vi "Ballistics_PBBA_beta.vi"() -> ()   [LabVIEW 2012]
doc: "This program is currently beta software. It is designed to address the data requirements defined primarily by the DHB Ballistic Test Report.\n\nThe general operation of this program is based on the Ballistics Version 2005 application developed internally by DuPont as a research tool for the Spruance Plant Ballistics Lab in Richmond, VA.\n\nPlease note that the original trigger control logic was modified and no longer depends on a safety interlock system to enable operation of a ballistic test.\n\nDuPont makes no warranties and assumes no liabilities in connection with any use of this program."
uses:
  <vilib>/Utility/NIReport.llb/NI_report.lvclass
  <vilib>/addons/database/NI_Database_API.lvlib
  <vilib>/addons/database/Connection.llb/Conn Execute.vi
  <vilib>/addons/database/Recordset.llb/Rec Destroy - Connection.vi
  <vilib>/Utility/config.llb/NI_LVConfig.lvlib
  <vilib>/Utility/config.llb/Write Key (I32).vi
  <vilib>/Analysis/NI_AALBase.lvlib
  Instance           1 28Saved   Ballistics_PBBA_beta .vi
  Shot Record.ctl
  <vilib>/addons/database/Connection.llb/DB Tools Open Connec (String).vi
  <vilib>/Utility/NIReport.llb/Append Text Table to Report (wrap).vi
  <vilib>/Utility/NIReport.llb/Append Report Text (str wrap).vi
panel:
  in  "RESET All":bool
  in  "EXIT":bool
  in  "Stop Program":bool
  in  "mainTabCntrl":enum32{"SETUP", "MEASURE", "HISTORY", "ABOUT"}(tab)
  in  "setupTabCntrl":T1(tab)
  in  "Model":u16(ring) caption="Model #" items=["n/a", "undefined", "other"]
  in  "clayCalArray":i16[](array[numeric])=[0, 0, 0, 0, 0] caption="Calibration" min=0 max=99 format="%02.0f"
  in  "Panel Dimensions":u16(ring)=6 caption="Panel Size" items=["7.5x7.5", "8.5x11", "12X12", "12x15", "13X13", "15X16", "15x15", "15x18", "16X16", "18X18", "20X16", "24x24", "101/4x113/4", "26X26", "CHEST PLATE", "HELMET", "VEST PANEL", "n/a"]
  out "threatDetails":T2
  in  "projectileWt":u16(ring) caption="Weight (gr)" items=["Select . . .", "2", "4", "16", "17", "44", "45", "55", "62", "64", "85", "110", "115", "123", "124", "127", "148", "158", "166", "180", "207", "240"]
  out "clayAverage":sgl caption="Clay Average" format="%#.1f"
  in  "clayTemp":i16 caption="Clay Temperature"
  in  "RoomT":i32 caption="Room Temperature"
  in  "RoomHum":i32 caption="Room Humidity"
  in  "Sample #":string
  in  "Comments":string caption="Remark"
  in  "recorder":u16(ring) caption="Recorder" items=["Mike Slate", "Dan Kraus", "Pat Fitzgerald", "Other"]
  in  "shooter":u16(ring) caption="Shooter" items=["Mike Slate", "Pat Fitzgerald", "Other"]
  in  "rangeNum":u16(ring) caption="Range #" items=["1", "2", "Other"]
  in  "projectileType":u16(ring) caption="Projectile Type"
  in  "weapon":u16(ring) caption="Weapon" items=["Universal Receiver", "Other"]
  in  "minV50":i32=1500 caption="Min. V50"
  in  "covering":u16(ring) caption="Ballistic Cover" items=["Other", "RipStop"]
  out "totalBAW":sgl caption="Total BAW" format="%.2f"
  in  "totalSampleWt":sgl caption="Total Weight" format="%.2f"
  in  "serialNum":string caption="Serial #"
  in  "workType":u16(ring) caption="Type of Work" items=["R&D", "QC", "Other"]
  in  "projNum":string caption="Project #"
  in  "projName":string caption="Project Name"
  in  "standard":u16(ring)=1 caption="Standard" items=["NIJ 0101.04", "MIL-STD-662F", "Other"]
  in  "Powder Type":u16(ring) items=["ACCURATE, NO. 2", "ACCURATE, NO. 9", "Alliant Herc. Bullseye", "Alliant 2400", "Hercules", "Hi-Skor 700x", "Hi-Skor 800x", "IMR-4198", "IMR-4756", "IMR-4895", "International Clay's", "Power Pistol", "Winchester Ball", "WINCHESTER-231", "WINCHESTER-296", "WINCHESTER-296"]
  in  "Method":u16(ring) items=["V50", "N.I.J.", "Quasi N.I.J.", "CUSUM", "V(0)", "V(0) @ 1450", "V(0) @ 1500", "V(0) @ 1550"]
  in  "Layer_1":T3={"plyNum"=0, "LotNum"="n/a", "RollNum"="n/a", "Fabric.stitch"=1} caption="Fabric #1" {"Fabric.stitch" items=["Corners", "Other", "n/a"]; "plyNum" min=0 max=99 step=5}
  in  "Layer_2":T3={"plyNum"=0, "LotNum"="n/a", "RollNum"="n/a", "Fabric.stitch"=1} caption="Fabric #2" {"Fabric.stitch" items=["Corners", "Other", "n/a"]; "plyNum" min=0 max=99 step=5}
  in  "Layer_3":T3={"plyNum"=0, "LotNum"="n/a", "RollNum"="n/a", "Fabric.stitch"=1} caption="Fabric #3" {"Fabric.stitch" items=["Corners", "Other", "n/a"]; "plyNum" min=0 max=99 step=5}
  in  "Layer_4":T3={"plyNum"=0, "LotNum"="n/a", "RollNum"="n/a", "Fabric.stitch"=1} caption="Fabric #4" {"Fabric.stitch" items=["Corners", "Other", "n/a"]; "plyNum" min=0 max=99 step=5}
  in  "Layer_5":T3={"plyNum"=0, "LotNum"="n/a", "RollNum"="n/a", "Fabric.stitch"=1} caption="Fabric #5" {"Fabric.stitch" items=["Corners", "Other", "n/a"]; "plyNum" min=0 max=99 step=5}
  in  "Layer_6":T3={"plyNum"=0, "LotNum"="n/a", "RollNum"="n/a", "Fabric.stitch"=1} caption="Fabric #6" {"Fabric.stitch" items=["Corners", "Other", "n/a"]; "plyNum" min=0 max=99 step=5}
  out "fabAttribs_1":T4 caption="fabricAttribs_1"
  out "fabAttribs_2":T4 caption="fabricAttribs_2"
  out "fabAttribs_3":T4 caption="fabricAttribs_3"
  out "fabAttribs_4":T4 caption="fabricAttribs_4"
  out "fabAttribs_5":T4 caption="fabricAttribs_5"
  out "fabAttribs_6":T4 caption="fabricAttribs_6"
  in  "fabStyle_1":u16(ring)
  in  "fabStyle_2":u16(ring)
  in  "fabStyle_3":u16(ring)
  in  "fabStyle_4":u16(ring)
  in  "fabStyle_5":u16(ring)
  in  "fabStyle_6":u16(ring)
  in  "fabVendor_1":u16(ring) caption="vendor" items=[" Select Vendor . . .", "Barrday", "Cushman", "DSM", "FMS", "Hexcell", "Honeywell", "Lincoln", "Pro Systems", "TEIJIN", "TexTech"]
  in  "fabVendor_2":u16(ring) caption="vendor" items=[" Select Vendor . . .", "Barrday", "Cushman", "DSM", "FMS", "Hexcell", "Honeywell", "Lincoln", "Pro Systems", "TEIJIN", "TexTech"]
  in  "fabVendor_3":u16(ring) caption="vendor" items=[" Select Vendor . . .", "Barrday", "Cushman", "DSM", "FMS", "Hexcell", "Honeywell", "Lincoln", "Pro Systems", "TEIJIN", "TexTech"]
  in  "fabVendor_4":u16(ring) caption="vendor" items=[" Select Vendor . . .", "Barrday", "Cushman", "DSM", "FMS", "Hexcell", "Honeywell", "Lincoln", "Pro Systems", "TEIJIN", "TexTech"]
  in  "fabVendor_5":u16(ring) caption="vendor" items=[" Select Vendor . . .", "Barrday", "Cushman", "DSM", "FMS", "Hexcell", "Honeywell", "Lincoln", "Pro Systems", "TEIJIN", "TexTech"]
  in  "fabVendor_6":u16(ring) caption="vendor" items=[" Select Vendor . . .", "Barrday", "Cushman", "DSM", "FMS", "Hexcell", "Honeywell", "Lincoln", "Pro Systems", "TEIJIN", "TexTech"]
  out "fab6_totalWt":sgl caption="Fab6 Wt" min=0 max=99 step=5 format="%.2f"
  out "fab5_totalWt":sgl caption="Fab5 Wt" min=0 max=99 step=5 format="%.2f"
  out "fab4_totalWt":sgl caption="Fab4 Wt" min=0 max=99 step=5 format="%.2f"
  out "fab3_totalWt":sgl caption="Fab3 Wt" min=0 max=99 step=5 format="%.2f"
  out "fab2_totalWt":sgl caption="Fab2 Wt" min=0 max=99 step=5 format="%.2f"
  out "fab1_totalWt":sgl caption="Fab1 Wt" min=0 max=99 step=5 format="%.2f"
  out "totalNumPlies":i32 caption="Total # of Plies" min=0 max=100 step=5
  in  "Next Shot":bool
  in  "Delete Button":bool
  in  "SHOTS":T5[](array[typedef]) {"UncorrectedAvgVel_PB" format="%.1f"; "strikeVel_PB" format="%.1f"; "velLoss_PB" format="%.1f"; "avgVel_PB" format="%.1f"; "Redundant_Velocity" format="%.1f"; "Energy Loss (J)" format="%.3e"; "Projectile Mass" min=0 step=1 format="%.4f"; "Corrected residual" format="%.2f"; "Uncorrected Residual" format="%.2f"; "Corrected Impact" format="%.2f"; "Uncorrected Impact" format="%.2f"; "Shot Angle" max=90 step=1; "SHOT STATUS" items=["Partial", "Complete"]; "IMPACT VELOCITY" min=0 max=10000 step=0.1 format="%.1f"; "Barrel Temperature" format="%.1f"; "Powder Loading" format="%.4f"; "RESIDUAL  VELOCITY" min=0 max=10000 step=0.1 format="%.1f"}
  in  "Refresh":bool
  in  "Clear":bool
  out "Shot":i32
  out "Panel":i32
  out "rangeOfResults":i32 caption="Range of Results" min=0 max=10000 step=1
  out "lowComplete":i32 caption="LOW Complete" min=0 max=10000 step=1
  out "highPartial":i32 caption="HIGH Partial" min=0 max=10000 step=1
  out "Avg/speed":sgl caption="Average" min=0 max=10000 step=0.1 format="%.1f"
  in  "Current/avg/speed":sgl caption="Average" min=0 max=1000000 step=0.1 format="%.1f"
  out "Redundant/speed":sgl caption="Chronograph 2" min=0 max=10000 step=0.1 format="%.1f"
  in  "backfacedia":sgl caption="BF Diameter"
  in  "backdepth":sgl caption="BF Depth"
  out "% Difference":sgl format="%.1f"
  out "zmr 2":sgl caption="Z.M.R." format="%.1f"
  out "Pairs":i16 min=0 max=100 step=1
  out "computed_V50":sgl caption="Value" format="%.1f"
  in  "maxDev":sgl=125.0 caption="Maximum\nDeviation" min=0 max=200 step=25 format="%.1f"
  in  "B.F.S (mm)":u16 caption="B.F.S"
  in  "N.I.J":u16(ring) items=["Not Tested", "PASS", "FAIL"]
  in  "Projectile Mass":sgl caption="Proj Mass (g)" min=0 step=1 format="%.4f"
  in  "Shot Angle":u16 max=90 step=1
  in  "Powder Loading":sgl min=0 max=100 step=0.1 format="%.3f"
  in  "Shot Decription":string
  in  "Barrel Temp":sgl format="%.1f"
  out "DC_ factor":sgl caption="Correction Factor (Mid-Chrono 1&2)" format="%.4f"
  in  "Current/redundant/speed":sgl caption="Chronograph 2" min=0 max=1000000 step=0.1 format="%.1f"
  out "currentDateTime":string caption="SUBMIT DATE/TIME"
  in  "Current/residual/speed":sgl caption="Residual" min=0 max=10000 step=0.1 format="%.1f"
  in  "Current/sthotstatus":u16(ring) caption="Penetration" items=["Partial", "Complete"]
  in  "Current/impact/speed":sgl caption="Chronograph 1" min=0 max=10000 step=0.1 format="%.1f"
  out "BACKFACE DEPTH":sgl caption="Backface\nDepth" min=0 max=200 step=5
  out "BACKFACE DIAMETER":sgl caption="Backface\nDiameter" min=0 max=100 step=5
  in  "Reject shot":bool
  in  "Accept Data":bool
  out "SUBMIT DATE/TIME":string
  out "residual/speed":sgl caption="Residual" min=0 max=10000 step=0.1 format="%.1f"
  out "SHOT STATUS":u16(ring) caption="Penetration" items=["Partial", "Complete"]
  out "Impact/speed":sgl caption="Chronograph 1" min=0 max=10000 step=0.1 format="%.1f"
  in  "Table of Shots":string[][](table) caption="Shot Table"
  in  "RANGE RESET":bool=TRUE caption="ARMED"
  in  "Save":bool
  in  "Report_PB":bool caption="Report"
  in  "Report Path":path=path "c:/ballistics"
  out "Data retrieval":string="\nWORKING"
  in  "historyTabCntrl":T6(tab)
  in  "Record #":i32=1 min=0 max=37
  in  "getRecord":bool
  out "Velocity versus Loading":cluster{dbl[], dbl[]}(graph)
  in  "Threat":string
  in  "Powder":string="bul"
  out "v50 data 2":string[][](table)
  in  "maxRecs":u16=1001 caption="Max # of Records" min=1 max=10000 step=100
  in  "Earliest Date":string="1/1/1990" caption="Begin Date"
  in  "velocity-loading":bool
  in  "latest Date":string="12/31/2010" caption="End Date"
  out "ActualNumRecs":i32=1001 caption="Actual # of Records Returned"
  out "Previous V50 Data":cluster{dbl, dbl, dbl[][]}(graph)={0.0, 1.0, []}
  out "v50 data":string[][](table)
  out "Average Velocity":dbl format="%.1f"
  out "CUSUM_lastVel":dbl caption="Latest Velocity" format="%.1f"
  out "CUSUM_stdDev":dbl caption="Std. Deviation" format="%.1f"
  in  "queryThreat":u16(ring) caption="Threat" items=["115-GRAIN,9mm LUGER,REFERENCE ROUND,10\" .38 cal TEST BBL.", "158-grain,WIN. 357 MAG, JHP REFERENCE ROUND, 10\" SAMMI TEST BBL.", "180-grain,WIN. 308 POWER-POINT REFERENCE ROUND, 308 TEST BBL.", "240-grain,REM. .44 mag, JSP REFERENCE ROUND, 8\" SAMMI TEST BBL."]
  out "In Control":bool=TRUE caption="Control Status"
  in  "Panel Search":bool
  in  "beginCUSUM":string="1/1/1900" caption="Begin Date"
  in  "endCUSUM":string="1/1/2100" caption="End Date"
  in  "aboutTabCntrl":T7(tab)
  out "Device S/N":string="DEVICE NOT READY!" caption="Timing Device S/N"
  in  "Data Source":u16(ring) items=["Simulated", "Radar", "Screens"]
  out "Distance Units":string="FEET"
  out "Weight Units":string="GRAMS"
  out "dbConn":string caption="Database Connection"
  in  "Sort by AVG":bool=TRUE caption="Sort shots by average velocity"
  in  "Add Disclaimer":bool
  in  "Report":bool
  out "Shot Graph":cluster{i32[], sgl[]}[](graph)
  out "Corrected Average":sgl=2206.6846 format="%.2f"
  out "Corrected Redundant":sgl=2256.401 format="%.2f"
  in  "mid_to_targ_dist":sgl=7.5 caption="Midpoint To Target Distance"
  out "conversion factor":sgl=0.3048037 format="%.5f"
  out "number of completes":i32=2
  out "number of partials":i32=2
  in  "percent warning":sgl=1.0 format="%.2f"
  in  "Version":dbl format="%.2f"
  out "impact/ID":u32=83886081 format="%.0x"
  out "residual/ID":u32=83951617 format="%.0x"
  out "Red/ID":u32=84017153 format="%.0x"
  out "correction coefficient":sgl=0.0252 format="%.8f"
  out "Corrected Residual":sgl=1210.3492 format="%.2f"
  out "Corrected Impact":sgl=2171.1157 format="%.2f"
  out "Impact/Separation":sgl=4.0 format="%.2f"
  out "Barrel to Screen":sgl=7.8333 format="%.2f"
  in  "Impact/Target Dist":sgl=7.083333 format="%.2f"
  out "Residual/Separation":sgl=4.0 format="%.2f"
  in  "Residual/Target Dist":sgl=7.083333 format="%.2f"
  out "Z.M.R.":sgl min=0 step=0.1 format="%.1f"
  in  "old threat":u16
  out "Complete":sgl[](array[numeric]) format="%.2f"
  out "factor array":sgl[](array[numeric])=[0.0252, 0.0191, 0.0191, 0.0441, 0.0425, 0.0131, 0.018] format="%.4f"
  out "Partial":sgl[](array[numeric]) format="%.2f"
  in  "DAQ Card":i16=1
  in  "Impact Timer":i16 min=0 max=3 step=1
  in  "Redundant Timer":i16=1 min=0 max=3 step=1
  in  "Residual  Timer":i16=2 min=0 max=3 step=1
  in  "Drag Corrected":bool
  out "Impact factor":sgl=0.94704616 caption="Impact" min=0 max=1 format="%.5f"
  out "Residual factor":sgl=1.0559148 caption="Residual" min=0 max=1 format="%.5f"
  in  "ballistician":u16(ring) caption="Ballistician" items=["Mike Slate", "Pat Fitzgerald"]
  in  "Threat 2":u16(ring) caption="Threat" items=["16 gr, saboted RCC,.308cal.SAAMI test bbl.,DC", "17 gr, saboted Type 1,FSP,.308cal. SAAMI test bbl.,DC", "17 gr, saboted Type 2,FSP,.308cal. SAAMI test bbl.,DC", "17 gr, saboted, STANAG 2920, FSP,.308 cal. SAMMI test bbl., DC", "2 gr, saboted RCC FSP,.223cal. SAAMI test bbl.,DC", "4 gr, saboted RCC FSP ,.223cal. SAAMI test bbl.,DC", "44 gr, 0.30-cal FSP - no sabot", "44 gr, saboted FSP,.458cal.SAAMI test bbl.,DC", "45 gr, JHP(WIN), .223 cal. SAMMI test bbl.", "55 gr, 0.223 M-193 FMJ  .223cal. SAAMI test bbl.", "62 gr, 0.223 M-855 Green Tip  .223cal SAAMI test bbl.", "64 gr, saboted RCC,.458cal.SAAMI test bbl.,DC"]
  in  "Panel Backing":u16(ring) items=["miscellaneous", "Clay (ROMA Plastilina # 1)", "Aluminum, 24 ga. (.020,.2024-T3) Witness Plate", "None"]
  in  "Submitter":u16(ring) items=["other"]
  in  "Test Conditions":u16(ring) items=["Dry", "Wet", "Hot 160 DEG. F", "Cold", "WEAPON LUBRICANT", "MOTOR OIL", "CONDITIONED", "ACCELERATED AGING"]
  in  "Panel Stitch":u16(ring)=5 items=["TEST PANEL/NORMAL STITCH", "TEST PANEL/CUSTOM STITCH", "VEST PANEL/CUSTOM STITCH", "HARD PANEL", "CAR ARMOR LAMINATE PANEL", "N.A."]
  in  "Panel Type":u16(ring)=4 items=["FABRIC ARMOR", "COMPOSITE ARMOR", "LG.RIGHT FRONT VEST PANEL", "HELMET", "N.A."]
  in  "Type":u16(ring) items=["none"]
  in  "Manufacturer":u16(ring)=1 caption="Mfr" items=["Point Blank-Marine Interceptor", "Other"]
  in  "Thickness":dbl format="%.2f"
  in  "Areal Density":dbl format="%.2f"
  in  "Areal density text":string
  in  "Fabric Description":string
  in  "Weight of Panel":dbl format="%.4f"
  in  "Panel Technician":u16(ring) items=["Not Known", "none", "POINT BLANK"]
  in  "clayCalib":string="##-##-##-##-##" caption="Calibration"
  in  "lookupRec":bool caption="lookup"
  out "connStr":string
  in  "message control":bool=TRUE
  # "yes"
  # "No"
  # "° F"
  # "%"
  # "° F"
  # "lbs"
  # "psf"
  # "mm"
  # "mm"
  # "in"
  # "GENERAL"
  # "SAMPLE"
  # "THREAT"
  # "RANGE"
  # "Fabric 1"
  # "Fabric 2"
  # "Fabric 3"
  # "Fabric 4"
  # "Fabric 5"
  # "Fabric 6"
  # "Vendor"
  # "Style #"
  # "# of Plies"
  # "Lot#"
  # "Roll#"
  # "Stitch"
  # "DHB ID#"
  # "Fiber"
  # "Denier"
  # "Pick"
  # "Weave"
  # "Finish"
  # "oz/yd²"
  # "Total Weight"
  # "STRIKE FACE -------------------------------------------------------- MODEL CONSTRUCTION -------------------------------------------------------- BODY SIDE"
  # "Edit any non-date field by placing cursor in field. \n\nProperties not listed are controlled by the current shot, test description or Fabric information.  \nIf the entry is changed for the current shot, then all previous shots are changed"
  # "V50"
  # "Current Shot Data"
  # "(mm)"
  # "Number of plies must be in FABRIC INFORMATION and SHOTS must exst in above table to enable saving"
  # "Last Assigned\nRecord Numbers"
  # "DuBAM\n\nDuPont Ballistics Automated Measurement\n\nPBBA Version 1.00\n\nDecember 2006"
  # "To arrange for technical support,\ncontact Pat Fitzgerald or Mark Hartsky\n\nDuPont Company"
  # "This software may be subject to revisions as additional experience and knowledge are gained. It is offered solely to provide possible suggestions for your own experimentation. It is not intended, however, to substitute for any testing you may need to conduct to determine for yourself the suitability of our software for your particular purposes. It is the user’s responsibility to determine the level of risk and the proper personal protection equipment needed. Because conditions are outside of our control, DUPONT MAKES NO WARRANTIES, EXPRESSED OR IMPLIED, AND ASSUMES NO LIABILITY WHATSOEVER AS TO THE PERFORMANCE OF THIS PRODUCT FOR A PARTICULAR USE. Nothing in this software is to be considered as a license to operate under or a recommendation to infringe any patent or trademark right. © 2006 E.I. du Pont de Nemours and Company. All rights reserved. DuPont™, the DuPont oval, the miracles of science®, KEVLAR ®, KEVLAR KM2 ®, are all trademarks or registered  trademarks of DuPont or its affiliates."
  # "Correction Factors"
  # "Yes"
  # "No"
  # "DuBAM"
  # "Version 1.00 for Point Blank Body Armor"
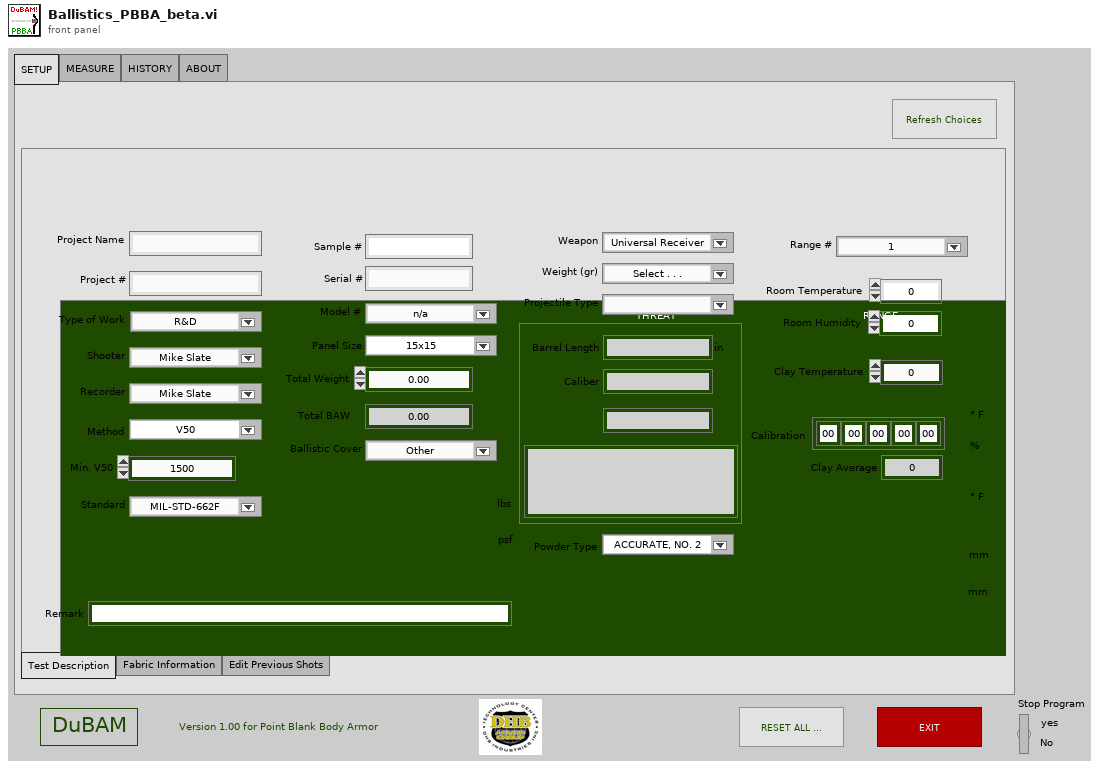
[diagram p1: front panel]
types:
  T1 = enum32{"Test Description", "Fabric Information", "Edit Previous Shots"}
  T2 = cluster{"barrelLength":string, "barrelCaliber":string, "dragCorrection":string, "detailDescription":string, "FK_threat":string}
  T3 = cluster{"plyNum":i32, "LotNum":string, "RollNum":string, "Fabric.stitch":u16}
  T4 = cluster{"Fabric.fiber":string, "Fabric.denier":string, "pick":string, "weave":string, "finish":string, "ozPerYd2":string, "fabricID_DHB":string, "SAK_fabric":string}
  T5 = typedef "Shot Record.ctl" = cluster{"avgVel_PB":sgl, "IMPACT VELOCITY":sgl, "RESIDUAL  VELOCITY ":sgl, "Shot Description":string, "Powder Loading ":sgl, "Barrel Temperature":sgl, "TIME / DATE":string, "shot order":i32, "SHOT STATUS":u16, "Shot Angle":u16, "Uncorrected Impact":sgl, "Corrected Impact":sgl, "Uncorrected Residual":sgl, "Corrected residual":sgl, "Projectile Mass":sgl, "usedv50":bool, "Energy Loss (J)":sgl, "BackFace\nDepth":sgl, "BackFace\nDiameter":sgl, "Redundant_Velocity":sgl, "velLoss_PB":sgl, "strikeVel_PB":sgl, "UncorrectedRed_PB":sgl, "CorrectedRed_PB":sgl, "UncorrectedAvgVel_PB":sgl}
  T6 = enum32{"Record Lookup", "Powder Loading", "CUSUM"}
  T7 = enum32{"About DuBAM", "NIJ Reference", "System", "Internal Use"}
  T8 = cluster{"impactCntrID":u32, "redundantCntrID":u32, "residualCntrID":u32}
  T9 = cluster{"Charset (-1)":i16, "Weight (-1)":i16, "Name":string, "Size":string}
  T10 = cluster{"Italic":enum16{"Italic Unchanged", "Italic On", "Italic Off"}, "Strike Through":enum16{"Strike Through Unchanged", "Strike Through On", "Strike Through Off"}, "Underline":enum16{"Underline Unchanged", "Underline On", "Underline Off"}, "Bold":enum16{"Bold Unchanged", "Bold On", "Bold Off"}}
  T11 = enum16{"Standard Report", "HTML", "Word", "Excel"}
  T12 = cluster{"[0]":string, "[1]":string, "[2]":string, "[3]":string, "[4]":string, "[5]":string, "[6]":string, "[7]":string, "[8]":string, "[9]":string}[]
  T13 = cluster{"plyNum":i32, "LotNum":string, "RollNum":string, "Fabric.stitch":u16}[]
  T14 = cluster{"Fabric.fiber":string, "Fabric.denier":string, "pick":string, "weave":string, "finish":string, "ozPerYd2":string, "fabricID_DHB":string, "SAK_fabric":string}[]
  T15 = cluster{string, string, string, string, string, string, string, string, "clayCalib":string, string}
  T16 = cluster{string, string, string, string, string, string, string}
  T17 = cluster{"Sample #":string, "element":string, "element":string, "serialNum":string, "element":string, string, string, string, "element":string, string}
  T18 = cluster{"[0]":string, "[1]":string, "[2]":string, "[3]":string, "[4]":string, "[5]":string, "[6]":string, "[7]":string, "[8]":string, "[9]":string}
  T19 = cluster{"element":string, "element":string, "element":string, "element":string, "barrelLength":string, string, "element":string, "element":string, "element":string}
  T20 = typedef "NI_Database_API.lvlib/Conn ObjectReference.ctl" = refnum<k1>
  T21 = typedef "NI_Database_API.lvlib/Rec ObjectReference.ctl" = refnum<k1>
  T22 = typedef "NI_LVConfig.lvlib/Config Data RefNum.ctl" = refnum<k1>
  T23 = cluster{"task ID out":u32, "task ID out":u32, "task ID out":u32}
  T24 = cluster{"fiber":string, "denier":string, "pick":string, "weave":string, "finish":string, "ozPerYd2":string, "fabricStyle_DHB":string, "fabricStyle_DHB 2":string}
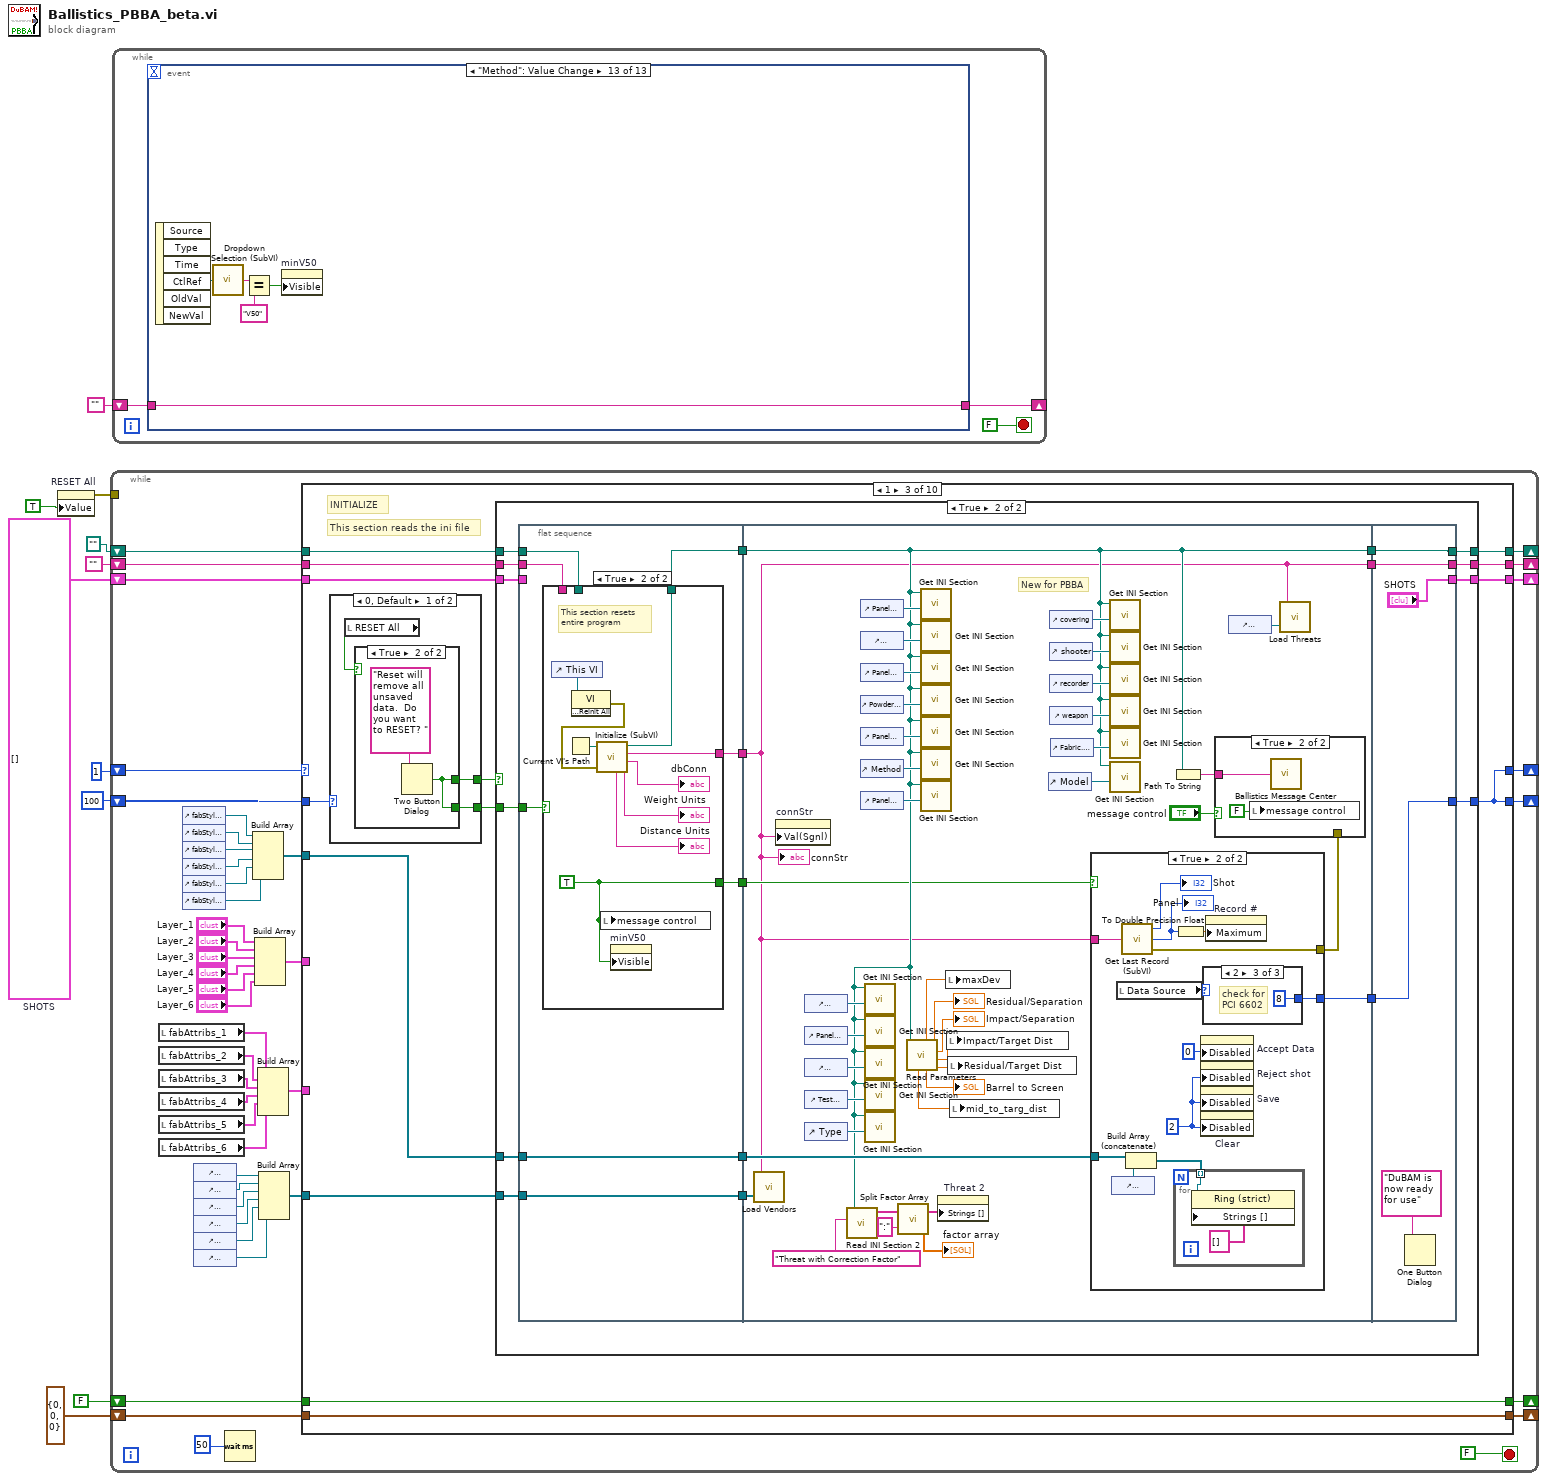
[diagram p0: block diagram]
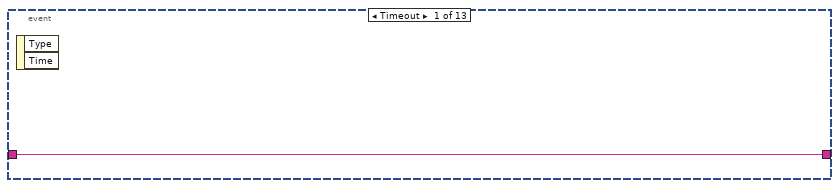
[diagram p2: hidden frame]
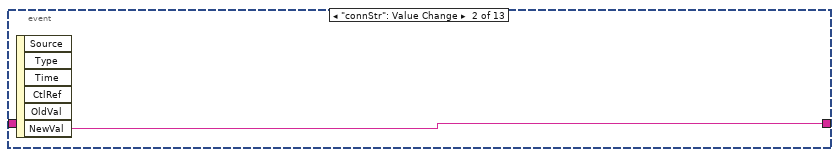
[diagram p3: hidden frame]
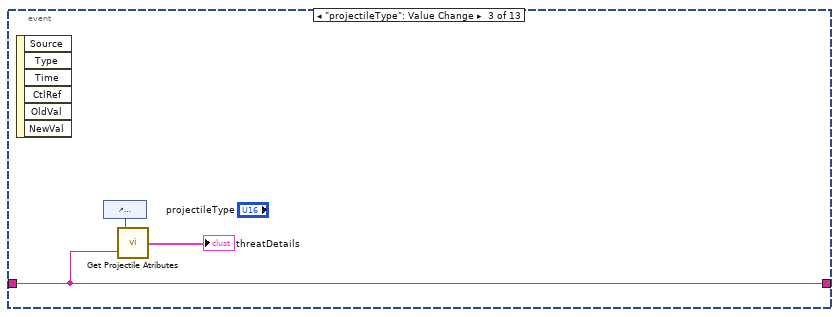
[diagram p4: hidden frame]
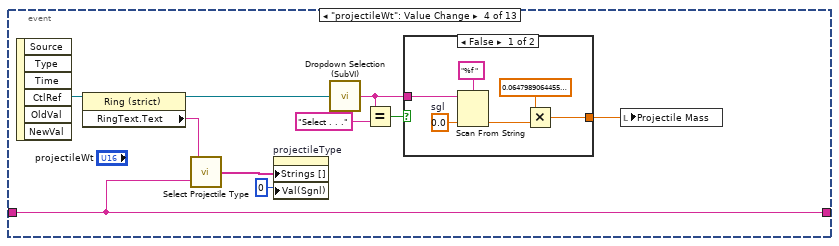
[diagram p5: hidden frame]
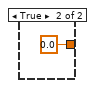
[diagram p6: hidden frame]
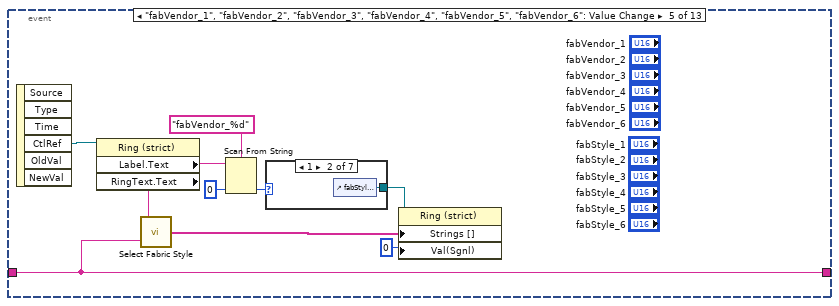
[diagram p7: hidden frame]
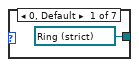
[diagram p8: hidden frame]
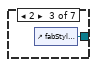
[diagram p9: hidden frame]
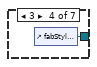
[diagram p10: hidden frame]
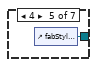
[diagram p11: hidden frame]
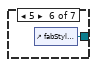
[diagram p12: hidden frame]
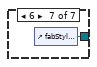
[diagram p13: hidden frame]
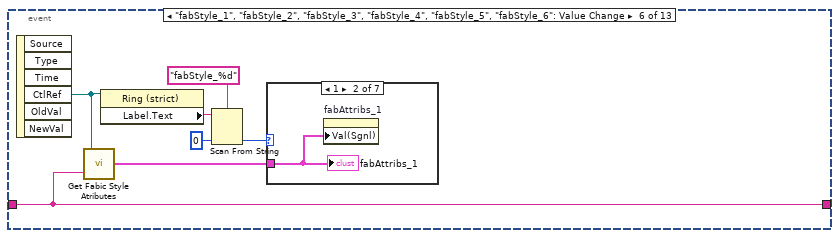
[diagram p14: hidden frame]
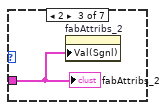
[diagram p16: hidden frame]
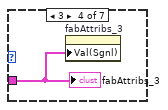
[diagram p17: hidden frame]
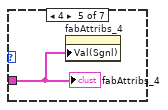
[diagram p18: hidden frame]
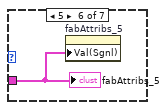
[diagram p19: hidden frame]
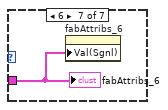
[diagram p20: hidden frame]
diagram:
  w4 = T5[] []  # SHOTS
  n1 = property on="RESET All" class="Bool (strict)"("Value"=TRUE ("RESET")) -> (error out=w7:errorcluster)  [unwired: 2 in, 1 out]
  n2 = while {
    shift-left: 100 -> [w50]
    shift-right: [w51] -> _
    shift-left: 1 ("index of element") -> [w54]
    shift-right: [w52] -> _
    tunnel: w7 -> [_]
    shift-right: [w48] -> _
    shift-left: T8 {"impactCntrID"=0, "redundantCntrID"=0, "residualCntrID"=0} -> [w47]
    shift-right: [w45] -> _
    shift-left: FALSE ("old drag") -> [w46]
    shift-right: [w43] -> _
    shift-left: w4 -> [w44]
    shift-right: [w14] -> _
    shift-left: path "" ("appended path OUT") -> [w13]
    shift-right: [w11] -> _
    shift-left: "" ("connectString") -> [w12]
    stop <- FALSE stop-if-true
    n3 = local read "fabAttribs_1"() -> (w42:T4)
    n4 = local read "fabAttribs_2"() -> (w40:T4)
    n5 = local read "fabAttribs_3"() -> (w39:T4)
    n6 = local read "fabAttribs_4"() -> (w38:T4)
    n7 = local read "fabAttribs_5"() -> (w37:T4)
    n8 = local read "fabAttribs_6"() -> (w41:T4)
    n9 = control-ref of="fabStyle_1"() -> (w21:refnum<vi>)
    n10 = control-ref of="fabStyle_2"() -> (w20:refnum<vi>)
    n11 = control-ref of="fabStyle_3"() -> (w19:refnum<vi>)
    n12 = control-ref of="fabStyle_4"() -> (w18:refnum<vi>)
    n13 = control-ref of="fabStyle_5"() -> (w17:refnum<vi>)
    n14 = control-ref of="fabStyle_6"() -> (w16:refnum<vi>)
    n15 = control-ref of="fabVendor_1"() -> (w28:refnum<vi>)
    n16 = control-ref of="fabVendor_2"() -> (w27:refnum<vi>)
    n17 = control-ref of="fabVendor_3"() -> (w26:refnum<vi>)
    n18 = control-ref of="fabVendor_4"() -> (w25:refnum<vi>)
    n19 = control-ref of="fabVendor_5"() -> (w24:refnum<vi>)
    n20 = control-ref of="fabVendor_6"() -> (w23:refnum<vi>)
    n21 = Wait (ms)(milliseconds to wait=u32 50 ("millisecond timer value")) -> ()  [unwired: 1 out]
    n22 = Build Array(w21, w20, w19, w18, w17, w16) -> (w15:refnum<vi>[])
    n23 = Build Array("Layer_1", "Layer_2", "Layer_3", "Layer_4", "Layer_5", "Layer_6") -> (w29:T13)
    n24 = Build Array(w42, w40, w39, w38, w37, w41) -> (w36:T14)
    n25 = Build Array(w28, w27, w26, w25, w24, w23) -> (w22:refnum<vi>[])
    n26 = case shown="1" w54 {
      tunnel: [w61 w454 w483 w748 w800 w1105 w1414 w1420 w1430 w1487] -> w52
      tunnel: [w62 w454 w483 w748 w800 w1104 w1414 w1420 w1430 w1487] -> w51
      tunnel: w50 -> [_ _ w486 _ _ _ _ _ _ _]
      tunnel: w44 -> [w63 w451 w480 w608 w763 w1093 w1375 _ w1428 w1479]
      tunnel: w13 -> [w56 w450 w485 w606 w765 w1095 w1373 w1416 w1424 w1478]
      tunnel: w12 -> [w55 w449 w484 w605 w764 w1094 w1372 w1415 w1423 w1477]
      tunnel: [w60 w453 w482 w626 w799 w1102 w1391 w1422 w1427 w1483] -> w48
      tunnel: w47 -> [w60 w453 w482 w626 w799 w1102 w1391 w1422 w1427 w1482]
      tunnel: w46 -> [w58 w452 w481 w609 w777 w1100 w1377 w1421 w1426 w1480]
      tunnel: [w59 w452 w481 w609 w777 w1100 w1376 w1421 w1426 w1480] -> w45
      tunnel: [w57 w451 w479 w608 w763 w1093 w1374 T5[] [] ("SHOTS") w1425 w1479] -> w43
      tunnel: w36 -> [_ _ _ _ w776 w1098 _ _ _ _]
      tunnel: w29 -> [_ _ _ _ w775 w1099 _ _ _ _]
      tunnel: w22 -> [_ _ w478 _ w774 w1096 _ _ _ _]
      tunnel: w15 -> [_ _ w477 _ w773 w1097 _ _ _ _]
      tunnel: [w56 w450 w476 w606 w765 w1095 w1373 w1416 w1424 w1478] -> w14
      tunnel: [w55 w449 w475 w605 w764 w1094 w1372 w1415 w1423 w1477] -> w11
      frame -1, Default {
        # "POLL"
        # "This section checks for any buttons, maintains routine check of the paramters"
        n27 = stacked-sequence {
          seq-local: [_ _ _ w330 _ _] -> [_ _ _ _ w364 _]
          seq-local: [_ _ w245 _ _ _] -> [_ _ _ w330 _ _]
          seq-local: [w66 _ _ _ _ _] -> [_ _ w222 _ _ _]
          tunnel: w63 -> [_ _ w221 _ w355 _]
          tunnel: [_ _ _ _ _ w420] -> w61
          tunnel: [_ _ _ _ _ -1] -> w62
          tunnel: w60 -> [w67 _ _ _ _ _]
          tunnel: [_ _ w223 _ _ _] -> w59
          tunnel: w58 -> [w65 _ _ _ _ _]
          tunnel: [_ _ _ _ w353 _] -> w57
          frame #0 {
            # "This section checks to see if the counters have been fired.  If they have then the counter times are read"
            n28 = local read "Data Source"() -> (w71:u16)
            n29 = Concatenate Strings("-1|", "F0|") -> (w68:string)
            n30 = case shown="0, Default" w71 {
              tunnel: [errorcluster {"status"=FALSE, "code"=0, "source"=""} ("error out") errorcluster {"status"=FALSE, "code"=0, "source"=""} ("error out") w116] -> w70
              tunnel: w68 -> [_ _ w112]
              tunnel: w67 -> [_ _ w108]
              tunnel: w65 -> [w73 w104 w107]
              tunnel: [w72 w104 w106] -> w66
              frame 0, Default {
                # "Simulated"
                n31 = local read "minV50"() -> (w77:i32)
                n32 = local read "Powder Loading"() -> (w97:sgl)
                n33 = To Single Precision Float(number=w77) -> (single precision float=w76:sgl)
                n34 = Not(x=w73) -> (.not. x?=w72:bool)
                n35 = call "Get Shell Speed.vi"("loading"=w97, "v50"=w76) -> ("impact"=w82:sgl, "residual"=w91:sgl)  [unwired: 2 in, 1 out]
                n36 = Random Number (0-1)() -> (number: 0 to 1=w89:dbl)
                n37 = To Single Precision Float(number=w89) -> (single precision float=w83:sgl)
                n38 = Multiply(x=w83, y=sgl 0.1) -> (x*y=w88:sgl)
                n39 = Add(x=w88, y=sgl 0.95) -> (x+y=w86:sgl)
                n40 = Greater Than 0?(x=w91) -> (x > 0?=w94:bool)
                n41 = Multiply(x=w82, y=w86) -> (x*y=w81:sgl)
                n42 = Add(x=w82, y=w81) -> (x+y=w79:sgl)
                n43 = Select(t=u16 1, s=w94, f=u16 0) -> (s? t:f=w92:u16)
                n44 = Divide(x=w79, y=sgl 2.0 ("v50")) -> (x/y=w78:sgl)
                n45 = local write "Current/impact/speed"(w82) -> ()
                n46 = local write "Current/residual/speed"(w91) -> ()
                n47 = local write "Current/redundant/speed"(w81) -> ()
                n48 = local write "SHOT STATUS"(w92) -> ()
                n49 = local write "Current/sthotstatus"(w92) -> ()
                n50 = local write "Current/avg/speed"(w78) -> ()
                n51 = Divide(x=sgl 2000.0, y=sgl 2.0 ("v50")) -> (x/y=w98:sgl)
                n52 = To Unsigned Long Integer(number=w98) -> (unsigned 32bit integer=w84:u32)
                n53 = local write "RANGE RESET"(TRUE ("RANGE RESET")) -> ()
                n54 = Wait (ms)(milliseconds to wait=w84) -> ()  [unwired: 1 out]
              }
              frame 1 {
                # "Radar -- (future)"
                n55 = local read "Current/redundant/speed"() -> (w99:sgl)
                n56 = local read "Current/impact/speed"() -> (w100:sgl)
                n57 = Add(x=w100, y=w99) -> (x+y=w102:sgl)
                n58 = Divide(x=w102, y=sgl 2.0) -> (x/y=w101:sgl)
                n59 = local write "Current/avg/speed"(w101) -> ()
              }
              frame 2 {
                # "Error -10600 occurrs in \"Read Count.vi\"\n\n  Possible reason(s):\n\n  NI-DAQ LV:\n    No setup operation has been performed for the specified resources. Or, some resources require a specific ordering of calls for proper setup.  \n\n  Solution: \n  To avoid this error, you must call the Dig_Line_Config function to setup the direction for each digital line prior to calling the Dig_Grp_Config function."
                # "Screens"
                n60 = Concatenate Strings(w112, "2|") -> (w111:string)
                n61 = Unbundle By Name(w108) -> ("impactCntrID"=w109:u32)
                n62 = call "Check Status.vi"("error in (no error)"=errorcluster {"status"=FALSE, "code"=0, "source"=""}, "TL Calling Location"=w111, "Task ID"=w109) -> ("error out"=w114:errorcluster, "Armed?"=w110:bool)  [unwired: 1 in]
                n63 = case shown="False" w110 {
                  tunnel: w114 -> [w142 w186]
                  tunnel: [w119 w186] -> w116
                  tunnel: w109 -> [w125 _]
                  tunnel: w111 -> [w138 _]
                  tunnel: w108 -> [w128 _]
                  tunnel: w107 -> [w118 w180]
                  tunnel: [w117 w180] -> w106
                  frame False {
                    n64 = local read "Impact/Separation"() -> (w145:sgl)
                    n65 = Concatenate Strings(w138, "F|") -> (w133:string)
                    n66 = Not(x=w118) -> (.not. x?=w117:bool)
                    n67 = call "Read Counter.vi"("TL Calling Location"=w133, "error In"=w142, "TASK ID"=w125) -> ("error out"=w127:errorcluster, "time (secs)"=w147:sgl)  [unwired: 3 in, 2 out]
                    n68 = Divide(x=w145, y=w147) -> (x/y=w121:sgl)
                    n69 = call "Arm One Channel.vi"("error IN"=w127, "task ID IN"=w125) -> ("error out"=w126:errorcluster)  [unwired: 2 in, 1 out]
                    n70 = Unbundle By Name(w128) -> ("redundantCntrID"=w130:u32)
                    n71 = Concatenate Strings(w133, "a|") -> (w136:string)
                    n72 = call "Check Status.vi"("error in (no error)"=w126, "TL Calling Location"=w136, "Task ID"=w130) -> ("error out"=w141:errorcluster, "Armed?"=w132:bool)  [unwired: 1 in]
                    n73 = case shown="False" w132 {
                      tunnel: [w158 sgl 0.0] -> w122
                      tunnel: w141 -> [w157 w162]
                      tunnel: [w152 w162] -> w143
                      tunnel: w130 -> [w151 _]
                      tunnel: w133 -> [w155 _]
                      frame False {
                        n74 = local read "Impact/Separation"() -> (w159:sgl)
                        n75 = Concatenate Strings(w155, "Fa|") -> (w154:string)
                        n76 = call "Read Counter.vi"("TL Calling Location"=w154, "error In"=w157, "TASK ID"=w151) -> ("error out"=w153:errorcluster, "time (secs)"=w160:sgl)  [unwired: 3 in, 2 out]
                        n77 = Divide(x=w159, y=w160) -> (x/y=w158:sgl)
                        n78 = call "Arm One Channel.vi"("error IN"=w153, "task ID IN"=w151) -> ("error out"=w152:errorcluster)  [unwired: 2 in, 1 out]
                      }
                      frame True {
                      }
                    }
                    n79 = Unbundle By Name(w128) -> ("residualCntrID"=w129:u32)
                    n80 = Concatenate Strings(w133, "b|") -> (w134:string)
                    n81 = call "Check Status.vi"("error in (no error)"=w143, "TL Calling Location"=w134, "Task ID"=w129) -> ("error out"=w140:errorcluster, "Armed?"=w131:bool)  [unwired: 1 in]
                    n82 = case shown="False" w131 {
                      tunnel: w140 -> [w169 w178]
                      tunnel: [w174 w179] -> w146
                      tunnel: w129 -> [w164 _]
                      tunnel: [w163 w178] -> w119
                      tunnel: [w171 sgl 0.0] -> w144
                      tunnel: w133 -> [w166 _]
                      frame False {
                        w175 = u16 1 items=["Partial", "Complete"] ("SHOT STATUS")
                        w176 = u16 0 items=["Partial", "Complete"] ("SHOT STATUS")
                        n83 = local read "Residual/Separation"() -> (w170:sgl)
                        n84 = Concatenate Strings(w166, "Fb|") -> (w167:string)
                        n85 = call "Read Counter.vi"("TL Calling Location"=w167, "error In"=w169, "TASK ID"=w164) -> ("error out"=w165:errorcluster, "counter overflow?"=w172:bool, "time (secs)"=w173:sgl)  [unwired: 3 in, 1 out]
                        n86 = Divide(x=w170, y=w173) -> (x/y=w171:sgl)
                        n87 = call "Arm One Channel.vi"("error IN"=w165, "task ID IN"=w164) -> ("error out"=w163:errorcluster)  [unwired: 2 in, 1 out]
                        n88 = Select(t=w176, s=w172, f=w175) -> (s? t:f=w174:u16)
                      }
                      frame True {
                        w179 = u16 1 items=["Partial", "Complete"] ("SHOT STATUS")
                      }
                    }
                    n89 = Add(x=w121, y=w122) -> (x+y=w123:sgl)
                    n90 = Divide(x=w123, y=sgl 2.0) -> (x/y=w120:sgl)
                    n91 = local write "Current/impact/speed"(w121) -> ()
                    n92 = local write "Current/redundant/speed"(w122) -> ()
                    n93 = local write "Current/residual/speed"(w144) -> ()
                    n94 = local write "Current/avg/speed"(w120) -> ()
                    n95 = local write "SHOT STATUS"(w146) -> ()
                    n96 = local write "Current/sthotstatus"(w146) -> ()
                    n97 = case shown="No Error" w119 {
                      selector: w119 -> [w150 _]
                      frame No Error {
                        n98 = Unbundle By Name(w150) -> ("status"=w149:bool)
                        n99 = Not(x=w149) -> (.not. x?=w148:bool)
                        n100 = local write "RANGE RESET"(w148) -> ()
                      }
                      frame Error {
                      }
                    }
                  }
                  frame True {
                    n101 = local read "Current/redundant/speed"() -> (w181:sgl)
                    n102 = local read "Current/impact/speed"() -> (w182:sgl)
                    n103 = Add(x=w182, y=w181) -> (x+y=w184:sgl)
                    n104 = Divide(x=w184, y=sgl 2.0) -> (x/y=w183:sgl)
                    n105 = local write "Current/avg/speed"(w183) -> ()
                  }
                }
              }
            }
            n106 = call <vilib>:"Simple Error Handler.vi"("error in (no error)"=w70) -> ()  [unwired: 4 in, 5 out]
          }
          frame #1 {
            n107 = local read "Current/impact/speed"() -> (w206:sgl)
            n108 = local read "Z.M.R."() -> (w209:sgl)
            n109 = local read "Current/redundant/speed"() -> (w207:sgl)
            n110 = Absolute Value(x=w209) -> (abs(x)=→"zmr 2":sgl)
            n111 = Add(x=w207, y=w206) -> (x+y=w205:sgl)
            n112 = Subtract(x=w207, y=w206) -> (x-y=w208:sgl)
            n113 = Divide(x=w205, y=sgl 200.0) -> (x/y=w204:sgl)
            n114 = Divide(x=w208, y=w204) -> (x/y=w200:sgl)
            "% Difference" <- w200
            n115 = Less Than 0?(x=w209) -> (x < 0?=w215:bool)
            n116 = Select(t="Lo C.- Hi P.", s=w215, f="Z.M.R.") -> (s? t:f=w212:string)
            n117 = Absolute Value(x=w200) -> (abs(x)=w197:sgl)
            n118 = Select(t=u32 65336, s=w215, f=u32 16755266) -> (s? t:f=w211:u32)
            n119 = Less?(x=w197, y="percent warning") -> (x < y?=w198:bool)
            n120 = property on="zmr 2" class="DigNum (strict)"("Caption.Text"=w212, "Numeric Text.Text Colors:BG Color"=w211) -> ()  [unwired: 2 in, 2 out]
            n121 = Select(t=u32 65343, s=w198, f=u32 15668992) -> (s? t:f=w196:u32)
            n122 = property on="% Difference" class="DigNum (strict)"("Numeric Text.Text Colors:BG Color"=w196) -> ()  [unwired: 2 in, 2 out]
            n123 = local read "Fabric Description"() -> (w193:string)
            n124 = local read "Shot Decription"() -> (w190:string)
            n125 = Get Date/Time In Seconds() -> (seconds since 1Jan1904=w187:timestamp)
            n126 = To Double Precision Float(number=w187) -> (double precision float=w217:dbl)
            n127 = String Subset(string=w193, length (rest)=75 ("length (rest)")) -> (substring=w192:string)  [unwired: 1 in]
            n128 = String Subset(string=w190, length (rest)=30 ("length (rest)")) -> (substring=w188:string)  [unwired: 1 in]
            n129 = local write "Fabric Description"(w192) -> ()
            n130 = local write "Shot Decription"(w188) -> ()
            n131 = Format Date/Time String(time format string (%c)="%x   %H:%M:%S", seconds (now)=w217) -> (date/time string=→"currentDateTime":string)  [unwired: 1 in]
            "BACKFACE DIAMETER" <- "backfacedia"
            "BACKFACE DEPTH" <- "backdepth"
          }
          frame #2 {
            n132 = disable-structure shown="Enabled" {
              disable-tunnel: "Threat 2" -> [w255 _]
              disable-tunnel: [w253 w259] -> w229
              frame Disabled {
                n133 = local read "factor array"() -> (w256:sgl[])
                n134 = To Long Integer(number=w255) -> (32bit integer=w254:i32)
                n135 = Index Array(array=w256, index=w254) -> (element=w253:sgl)
              }
              frame Enabled {
                n136 = local read "threatDetails"() -> (w257:T2)
                n137 = Unbundle By Name(w257) -> ("dragCorrection"=w258:string)
                n138 = Scan From String(input string=w258, default 1=sgl 0.0 ("default value 1")) -> (output 1=w259:sgl)  [unwired: 3 in, 3 out]
              }
            }
            "correction coefficient" <- w229
            n139 = local read "Distance Units"() -> (w231:string)
            n140 = call "Compute Strike Velocity.vi"("drag coefficient"=w229, "decay distance"="mid_to_targ_dist", "raw velocity"="Current/avg/speed", "distance units"=w231) -> ("correction factor"=w224:sgl, "strike velocity"=w225:sgl)  [unwired: 1 out]
            "DC_ factor" <- w224
            "Corrected Average" <- w225
            n141 = call "Velocity Correction.vi"("raw impact"="Current/impact/speed", "distance units"=w231, "raw redundant"="Current/redundant/speed", "raw residual"="Current/residual/speed", "screen set midpt to target"="Impact/Target Dist", "residual screen to target"="Residual/Target Dist", "correction coefficient"=w229) -> ("corrected impact"=w241:sgl, "corrected redundant"=w234:sgl, "corrected residual"=w239:sgl, "impact factor"=w237:sgl, "conversion factor"=→"conversion factor":sgl, "residual factor"=w236:sgl)  [unwired: 3 in]
            "Residual factor" <- w236
            "Impact factor" <- w237
            "Corrected Impact" <- w241
            "Corrected Residual" <- w239
            "Corrected Redundant" <- w234
            n142 = Not Equal?(x="Drag Corrected", y=w222) -> (x != y?=w247:bool)
            n143 = Select(t=w234, s="Drag Corrected", f="Current/redundant/speed") -> (s? t:f=→"Redundant/speed":sgl)
            n144 = Select(t=w225, s="Drag Corrected", f="Current/avg/speed") -> (s? t:f=→"Avg/speed":sgl)
            n145 = Select(t=w241, s="Drag Corrected", f="Current/impact/speed") -> (s? t:f=→"Impact/speed":sgl)
            n146 = Select(t=w239, s="Drag Corrected", f="Current/residual/speed") -> (s? t:f=→"residual/speed":sgl)
            n147 = Not Equal?(x="Threat 2", y="old threat") -> (x != y?=w248:bool)
            n148 = Or(x=w248, y=w247) -> (x .or. y?=w246:bool)
            n149 = case shown="True" w246 {
              tunnel: "Threat 2" -> [_ w269]
              tunnel: w221 -> [w262 w268]
              tunnel: w236 -> [_ w267]
              tunnel: w237 -> [_ w266]
              tunnel: "Drag Corrected" -> [w261 w263]
              tunnel: [w262 w265] -> w245
              tunnel: w224 -> [_ w264]
              tunnel: [w261 w263] -> w223
              frame False {
              }
              frame True {
                n150 = local write "old threat"(w269) -> ()
                n151 = for {
                  tunnel: w268 -> [w285] mode=indexing
                  tunnel: w267 -> [w295]
                  tunnel: w266 -> [w290]
                  tunnel: w263 -> [w282]
                  tunnel: [w297] -> w265 mode=indexing
                  tunnel: w264 -> [w283]
                  n152 = Unbundle By Name(w285) -> ("UncorrectedAvgVel_PB"=w284:sgl)
                  n153 = Unbundle By Name(w285) -> ("Uncorrected Impact"=w289:sgl)
                  n154 = Unbundle By Name(w285) -> ("Uncorrected Residual"=w294:sgl)
                  n155 = Unbundle By Name(w285) -> ("UncorrectedRed_PB"=w292:sgl)
                  n156 = Multiply(x=w283, y=w284) -> (x*y=w280:sgl)
                  n157 = Multiply(x=w290, y=w292) -> (x*y=w291:sgl)
                  n158 = Multiply(x=w290, y=w289) -> (x*y=w287:sgl)
                  n159 = Multiply(x=w295, y=w294) -> (x*y=w286:sgl)
                  n160 = Select(t=w280, s=w282, f=w284) -> (s? t:f=w281:sgl)
                  n161 = Select(t=w291, s=w282, f=w292) -> (s? t:f=w293:sgl)
                  n162 = Select(t=w286, s=w282, f=w294) -> (s? t:f=w296:sgl)
                  n163 = Select(t=w287, s=w282, f=w289) -> (s? t:f=w288:sgl)
                  n164 = Subtract(x=w281, y=w280) -> (x-y=w279:sgl)
                  n165 = Bundle By Name(cluster=w285, "velLoss_PB"=w279, "strikeVel_PB"=w280, "avgVel_PB"=w281, "CorrectedRed_PB"=w291, "Redundant_Velocity"=w293, "Corrected Impact"=w287, "IMPACT VELOCITY"=w288, "Corrected residual"=w286, "RESIDUAL  VELOCITY"=w296) -> (w297:T5)
                }
                n166 = disable-structure shown="Disabled" {
                  frame Disabled {
                    w270 = sgl 0.0  # sgl
                    n167 = property on="Threat 2" class="Ring (strict)"() -> ("Strings []"=w278:string[], "Value"=w277:u16)  [unwired: 2 in, 2 out]
                    n168 = To Long Integer(number=w277) -> (32bit integer=w272:i32)
                    n169 = Index Array(array=w278, index=w272) -> (element=w276:string)
                    n170 = Scan From String(format string="%f " ("Format String"), input string=w276, default 1=w270) -> (output 1=w271:sgl)  [unwired: 2 in, 3 out]
                    n171 = Multiply(x=sgl 0.06479891, y=w271) -> (x*y=w273:sgl)
                    n172 = local write "Projectile Mass"(w273) -> ()
                  }
                  frame Enabled {
                  }
                }
              }
            }
            "SHOT STATUS" <- "Current/sthotstatus"
          }
          frame #3 {
            w298 = sgl[] [] ("Partial")
            # "This section calculates the V50"
            n173 = local read "totalNumPlies"() -> (w326:i32)
            n174 = Array Size(array=w330) -> (size(s)=w329:i32)
            n175 = Equal To 0?(x=w329) -> (x = 0?=w319:bool)
            n176 = Equal To 0?(x=w326) -> (x = 0?=w325:bool)
            n177 = Or(x=w319, y=w325) -> (x .or. y?=w324:bool)
            n178 = Select(t=u8 2, s=w319, f=u8 0) -> (s? t:f=w320:u8)
            n179 = Select(t=u8 2, s=w324, f=u8 0) -> (s? t:f=w323:u8)
            n180 = property on="Save" class="Bool"("Disabled"=w323) -> ()  [unwired: 2 in, 2 out]
            n181 = property on="Clear" class="Bool"("Disabled"=w320) -> ()  [unwired: 2 in, 2 out]
            n182 = for {
              shift-right: [w339] -> w301
              shift-left: w298 -> [w340]
              shift-right: [w337] -> w300
              shift-left: w298 -> [w338]
              tunnel: w330 -> [w335] mode=indexing
              shift-right: [w333] -> w299
              shift-left: w298 -> [w332]
              # "Here, DuPont uses:\n\nIMPACT VELOCITY"
              n183 = Unbundle By Name(w335) -> ("strikeVel_PB"=w331:sgl, "SHOT STATUS"=w336:u16)
              n184 = Unbundle By Name(w335) -> ("usedv50"=w334:bool)
              n185 = case shown="True" w334 {
                tunnel: [w341 w344] -> w333
                tunnel: w332 -> [w341 w343]
                tunnel: w331 -> [_ w342]
                frame False {
                }
                frame True {
                  n186 = Build Array (concatenate)(w343, w342) -> (w344:sgl[])
                }
              }
              n187 = case shown="0, Default" w336 {
                tunnel: w331 -> [w345 w349]
                tunnel: [w348 w350] -> w339
                tunnel: w340 -> [w347 w350]
                tunnel: w338 -> [w346 w352]
                tunnel: [w346 w351] -> w337
                frame 0, Default {
                  n188 = Build Array (concatenate)(w347, w345) -> (w348:sgl[])
                }
                frame 1 {
                  n189 = Build Array (concatenate)(w352, w349) -> (w351:sgl[])
                }
              }
            }
            n190 = Sort 1D Array(array=w301) -> (sorted array=w318:sgl[])
            n191 = Sort 1D Array(array=w300) -> (sorted array=w306:sgl[])
            "Complete" <- w306
            n192 = Array Max & Min(array=w299) -> (max value=w310:sgl, min value=w309:sgl)  [unwired: 2 out]
            n193 = Array Size(array=w306) -> (size(s)=→"number of completes":i32)
            n194 = Reverse 1D Array(array=w318) -> (reversed array=w304:sgl[])
            "Partial" <- w304
            n195 = Array Max & Min(array=w306) -> (min value=w312:sgl)  [unwired: 3 out]
            n196 = Subtract(x=w310, y=w309) -> (x-y=w308:sgl)
            n197 = Array Size(array=w304) -> (size(s)=→"number of partials":i32)
            n198 = Array Max & Min(array=w304) -> (max value=w314:sgl)  [unwired: 3 out]
            n199 = call "Compute V50.vi"("Maximum Deviation"="maxDev", "Partial"=w304, "Complete"=w306) -> ("zmr"=→"Z.M.R.":sgl, "Points"=→"Pairs":i16, "V50"=→"computed_V50":sgl)
            n200 = To Long Integer(number=w308) -> (32bit integer=→"rangeOfResults":i32)
            n201 = To Long Integer(number=w314) -> (32bit integer=→"highPartial":i32)
            n202 = To Long Integer(number=w312) -> (32bit integer=→"lowComplete":i32)
          }
          frame #4 {
            n203 = local read "Pairs"() -> (w361:i16)
            n204 = Sort 1D Array(array=w364) -> (sorted array=w358:T5[])
            n205 = for {
              tunnel: w358 -> [w409] mode=indexing
              tunnel: w361 -> [w400]
              shift-right: [w399] -> _
              shift-left: i16 0 -> [w398]
              tunnel: [w392] -> w359 mode=indexing
              # "this section marks the lowest completes that are used in V50"
              n206 = Unbundle By Name(w409) -> ("SHOT STATUS"=w396:u16, "Projectile Mass"=w394:sgl, "avgVel_PB"=w393:sgl, "RESIDUAL  VELOCITY"=w395:sgl)
              n207 = local read "conversion factor"() -> (w402:sgl)
              n208 = case shown="1" w396 {
                tunnel: w400 -> [_ w416]
                tunnel: [FALSE w415] -> w397
                tunnel: [w411 w414] -> w399
                tunnel: w398 -> [w411 w412]
                frame 0, Default {
                }
                frame 1 {
                  n209 = Less?(x=w412, y=w416) -> (x < y?=w415:bool)
                  n210 = Add(x=w412, y=i16 1 ("t")) -> (x+y=w414:i16)
                }
              }
              n211 = Multiply(x=w402, y=w395) -> (x*y=w403:sgl)
              n212 = Multiply(x=w393, y=w402) -> (x*y=w404:sgl)
              n213 = Multiply(x=w404, y=w404) -> (x*y=w408:sgl)
              n214 = Multiply(x=w403, y=w403) -> (x*y=w407:sgl)
              n215 = Subtract(x=w408, y=w407) -> (x-y=w406:sgl)
              n216 = Compound Arithmetic op=MULTIPLY(w394, w406, sgl 0.0005 ("Input")) -> (w401:sgl)
              n217 = Bundle By Name(cluster=w409, "usedv50"=w397, "Energy Loss (J)"=w401) -> (w392:T5)
            }
            n218 = Reverse 1D Array(array=w359) -> (reversed array=w357:T5[])
            n219 = for {
              tunnel: w357 -> [w369] mode=indexing
              tunnel: w361 -> [w372]
              shift-right: [w370] -> _
              shift-left: i16 0 -> [w371]
              tunnel: [w367] -> w354 mode=indexing
              # "chooses highest partials used in v50"
              n220 = Unbundle By Name(w369) -> ("SHOT STATUS"=w373:u16, "usedv50"=w366:bool)
              n221 = case shown="0, Default" w373 {
                tunnel: w372 -> [w377 _]
                tunnel: [w376 w380] -> w368
                tunnel: w371 -> [w374 w379]
                tunnel: [w375 w379] -> w370
                tunnel: w366 -> [_ w380]
                frame 0, Default {
                  n222 = Less?(x=w374, y=w377) -> (x < y?=w376:bool)
                  n223 = Add(x=w374, y=i16 1) -> (x+y=w375:i16)
                }
                frame 1 {
                }
              }
              n224 = Bundle By Name(cluster=w369, "usedv50"=w368) -> (w367:T5)
            }
            n225 = case shown="True" "Next Shot" {
              tunnel: w354 -> [w381 w383]
              tunnel: [w381 w382] -> w353
              frame False {
              }
              frame True {
                n226 = property on="SHOTS" class="Arr (strict)"() -> ("Index Values"=w385:u32[])  [unwired: 2 in, 2 out]
                n227 = local write "Next Shot"(FALSE ("Boolean")) -> ()
                n228 = Array Size(array=w383) -> (size(s)=w388:i32)
                n229 = Index Array(array=w385) -> (element=w390:u32)  [unwired: 1 in]
                n230 = To Unsigned Long Integer(number=w388) -> (unsigned 32bit integer=w384:u32)
                n231 = Increment(x=w390) -> (x+1=w389:u32)
                n232 = Quotient & Remainder(x=w389, y=w384) -> (x-y*floor(x/y)=w387:u32)  [unwired: 1 out]
                n233 = Replace Array Subset(array=w385, new element=w387) -> (w386:u32[])  [unwired: 1 in]
                n234 = property on="SHOTS" class="Arr (strict)"("Index Values"=w386) -> ("Value"=w382:T5[])  [unwired: 2 in, 2 out]
              }
            }
            n235 = Not Equal?(x=w355, y=w353) -> (x != y?=w356:bool)
            n236 = case shown="True" w356 {
              tunnel: w353 -> [_ w365]
              frame False {
              }
              frame True {
                n237 = property on="SHOTS" class="Arr (strict)"("Val(Sgnl)"=w365) -> ()  [unwired: 2 in, 2 out]
              }
            }
          }
          frame #5 {
            w429 = TRUE  # element
            n238 = Or(x="RESET All", y="Refresh") -> (x .or. y?=w438:bool)
            n239 = Or(x="Report_PB", y="getRecord") -> (x .or. y?=w418:bool)
            n240 = Or(x="Reject shot", y="Delete Button") -> (x .or. y?=w433:bool)
            n241 = case shown="True" "Stop Program" {
              frame False {
              }
              frame True {
                n242 = Stop() -> ()  [unwired: 1 in]
              }
            }
            n243 = Build Array("EXIT", w438, "Report", w418, "Save", "Accept Data", "Clear", w433, "RANGE RESET") -> (w428:bool[])
            n244 = Search 1D Array(1D array=w428, element=w429) -> (index of element=w421:i32)  [unwired: 1 in]
            n245 = Equal?(x=w421, y=4) -> (x = y?=w422:bool)
            n246 = case shown="False" w422 {
              tunnel: w421 -> [w440 w441]
              tunnel: [w440 w446] -> w420
              frame False {
              }
              frame True {
                # "Before allowing data record to be saved,\nprompt user to validate."
                n247 = Two Button Dialog(message="Are ALL Data Valid?", 1:"NO" ("F button name (\"Cancel\")"), 2:"YES" ("T button name (\"OK\")")) -> (T button?=w445:bool)
                n248 = case shown="False" w445 {
                  tunnel: [-1 ("index of element") w448] -> w446
                  tunnel: w441 -> [_ w448]
                  frame False {
                  }
                  frame True {
                  }
                }
              }
            }
          }
        }
      }
      frame 0 {
        w454 = -1 ("index of element")
        # "Apparently dead or unreachable code"
        # "EXIT"
        # "This section stops program"
        n249 = disable-structure shown="Disabled" {
          disable-tunnel: w451 -> [w457 _]
          frame Disabled {
            # "SET PENETRATION STATUS"
            # "This section is supposed to switch the setting from partial to complete"
            n250 = Array Size(array=w457) -> (size(s)=w467:i32)
            n251 = Decrement(x=w467) -> (x-1=w459:i32)
            n252 = Index Array(array=w457, index=w459) -> (element=w462:T5)
            n253 = Unbundle By Name(w462) -> ("SHOT STATUS"=w466:u16)
            n254 = Equal To 0?(x=w466) -> (x = 0?=w465:bool)
            n255 = Select(t=u16 1, s=w465, f=u16 0) -> (s? t:f=w461:u16)
            n256 = local write "Current/sthotstatus"(w461) -> ()
            n257 = Bundle By Name(cluster=w462, "SHOT STATUS"=w461) -> (w460:T5)
            n258 = Replace Array Subset(array=w457, new element=w460, index=w459) -> (w458:T5[])
            n259 = stacked-sequence {
              tunnel: w461 -> [_]
              tunnel: w458 -> [w468]
              frame #0 {
                n260 = call "Update Shot Table.vi"("shot array"=w468) -> ("shotTable OUT"=w469:string[][])
                n261 = local write "Table of Shots"(w469) -> ()
                n262 = local write "SHOTS"(w468) -> ()
              }
            }
          }
          frame Enabled {
          }
        }
        n263 = Two Button Dialog(message="All Unsaved data will be lost.   Do you want to quit the program? ") -> (T button?=w456:bool)  [unwired: 2 in]
        n264 = case shown="True" w456 {
          frame False {
          }
          frame True {
            n265 = Quit LabVIEW(quit? (T)=TRUE) -> ()
          }
        }
        n266 = disable-structure shown="Disabled" {
          frame Disabled {
            # "DUPONT CONTACT SHOT REPORT (Unused)"
            # "This section prepares a Contact Shot report"
            n267 = control-ref of="Shot Graph"() -> (w472:refnum<vi>)
            n268 = control-ref of="Sample #"() -> (w471:refnum<vi>)
            n269 = control-ref of="Report Path"() -> (w470:refnum<vi>)
            n270 = call "Contact Report (SubVI).vi"("reportPath_ref"=w470, "SampleIDref"=w471, "Shot Graph"=w472) -> ()
          }
          frame Enabled {
          }
        }
      }
      frame 1 {
        # "INITIALIZE"
        # "This section reads the ini file"
        n271 = case shown="0, Default" w486 {
          tunnel: [w490 w495] -> w487
          tunnel: [w488 w495] -> w474
          frame 0, Default {
            n272 = local read "RESET All"() -> (w489:bool)
            n273 = case shown="True" w489 {
              tunnel: [TRUE w493] -> w490
              tunnel: [FALSE w493] -> w488
              frame False {
                # "Refresh"
              }
              frame True {
                n274 = Two Button Dialog(message="Reset will remove all unsaved data.  Do you want to RESET? ") -> (T button?=w493:bool)  [unwired: 2 in]
              }
            }
          }
          frame 100 {
            w495 = TRUE
          }
        }
        n275 = case shown="True" w487 {
          tunnel: w485 -> [w497 w518]
          tunnel: w484 -> [w496 w517]
          tunnel: [-1 ("index of element") w516] -> w483
          tunnel: w480 -> [w498 w514]
          tunnel: [w498 w513] -> w479
          tunnel: w478 -> [_ w512]
          tunnel: w477 -> [_ w511]
          tunnel: [w497 w506] -> w476
          tunnel: [w496 w503] -> w475
          tunnel: w474 -> [_ w501]
          frame False {
            n276 = local write "RESET All"(FALSE ("RESET")) -> ()
          }
          frame True {
            n277 = flat-sequence {
              tunnel: w511 -> [w525]
              tunnel: w512 -> [w526]
              tunnel: w514 -> [_]
              tunnel: w517 -> [w520]
              tunnel: w518 -> [w523]
              tunnel: [w522] -> w510
              tunnel: [w526] -> w509
              tunnel: [w525] -> w508
              tunnel: w501 -> [w524]
              tunnel: [w521] -> w505
              tunnel: [w519] -> w502
              tunnel: [w567] -> w515
              tunnel: w510 -> [w541]
              tunnel: w509 -> [w546]
              tunnel: w508 -> [w543]
              tunnel: [w541] -> w507
              tunnel: w505 -> [w539]
              tunnel: [w539] -> w504
              tunnel: w502 -> [w540]
              tunnel: [w604] -> w516
              tunnel: w515 -> [w604]
              tunnel: ["SHOTS"] -> w513
              tunnel: [w601] -> w506
              tunnel: w507 -> [w601]
              tunnel: [w600] -> w503
              tunnel: w504 -> [w600]
              frame #0 {
                n278 = case shown="True" w524 {
                  tunnel: [w529 w533] -> w522
                  tunnel: w523 -> [w529 _]
                  tunnel: [w528 w532] -> w521
                  tunnel: w520 -> [w528 _]
                  tunnel: [w527 w530] -> w519
                  frame False {
                    w527 = FALSE  # Reset All
                    # "Refresh"
                  }
                  frame True {
                    w530 = TRUE
                    # "This section resets\nentire program"
                    n279 = control-ref of="This VI"() -> (w538:refnum<vi>)
                    n280 = Current VI's Path() -> (path=w537:path)
                    n281 = invoke class="VI" method="Default Vals.Reinit All"(reference=w538) -> (error out=w531:errorcluster)  [unwired: 2 in, 2 out]
                    n282 = call "Initialize (SubVI).vi"(5:w537, "error IN"=w531) -> ("appended path OUT"=w533:path, "connectString"=w532:string, "Database Connection"=→"dbConn":string, "Weight Units"=→"Weight Units":string, "Distance Units"=→"Distance Units":string)  [unwired: 1 in]
                    n283 = local write "message control"(w530) -> ()
                    n284 = property on="minV50" class="DigNum (strict)"("Visible"=w530) -> ()  [unwired: 2 in, 2 out]
                  }
                }
              }
              frame #1 {
                # "New for PBBA"
                n285 = call "Load Vendors.vi"("Vendor array"=w546, "connectString"=w539) -> ()  [unwired: 1 out]
                n286 = property on="connStr" class="Str"("Val(Sgnl)"=w539) -> ()  [unwired: 2 in, 2 out]
                n287 = control-ref of="ballistician"() -> (w558:refnum<vi>)
                n288 = control-ref of="Panel Technician"() -> (w557:refnum<vi>)
                n289 = control-ref of="Manufacturer"() -> (w556:refnum<vi>)
                n290 = control-ref of="Test Conditions"() -> (w555:refnum<vi>)
                n291 = control-ref of="Type"() -> (w554:refnum<vi>)
                n292 = call "Read INI Section 2.vi"("section"="Threat with Correction Factor", "configuration file path"=w541) -> ("Array"=w577:string[])  [unwired: 4 in, 1 out]
                n293 = control-ref of="Panel Backing"() -> (w547:refnum<vi>)
                n294 = control-ref of="Submitter"() -> (w548:refnum<vi>)
                n295 = control-ref of="Panel Dimensions"() -> (w549:refnum<vi>)
                n296 = control-ref of="Powder Type"() -> (w550:refnum<vi>)
                n297 = control-ref of="Panel Type"() -> (w551:refnum<vi>)
                n298 = control-ref of="Method"() -> (w552:refnum<vi>)
                n299 = control-ref of="Panel Stitch"() -> (w553:refnum<vi>)
                n300 = call "Get INI Section.vi"("Ring Refnum"=w558, "configuration file path"=w541) -> ()  [unwired: 4 in, 2 out]
                n301 = call "Get INI Section.vi"("Ring Refnum"=w557, "configuration file path"=w541) -> ()  [unwired: 4 in, 2 out]
                n302 = call "Get INI Section.vi"("Ring Refnum"=w556, "configuration file path"=w541) -> ()  [unwired: 4 in, 2 out]
                n303 = call "Get INI Section.vi"("Ring Refnum"=w555, "configuration file path"=w541) -> ()  [unwired: 4 in, 2 out]
                n304 = call "Get INI Section.vi"("Ring Refnum"=w554, "configuration file path"=w541) -> ()  [unwired: 4 in, 2 out]
                n305 = call "Split Factor Array.vi"("Split character"=":", "STRING INPUT"=w577) -> ("FACTOR OUTPUT"=→"factor array":sgl[], "STRING OUTPUT"=w575:string[])
                n306 = call "Read Parameters.vi"("appended path"=w541) -> ("midpt_to_target_dist"=w563:sgl, "max dev"=w571:sgl, "residual separation"=→"Residual/Separation":sgl, "impact separation"=→"Impact/Separation":sgl, "barrel screen dist"=→"Barrel to Screen":sgl, "impact target dist"=w570:sgl, "resid target dist"=w569:sgl)  [unwired: 3 in]
                n307 = call "Get INI Section.vi"("Ring Refnum"=w547, "configuration file path"=w541) -> ()  [unwired: 4 in, 2 out]
                n308 = call "Get INI Section.vi"("Ring Refnum"=w548, "configuration file path"=w541) -> ()  [unwired: 4 in, 2 out]
                n309 = call "Get INI Section.vi"("Ring Refnum"=w549, "configuration file path"=w541) -> ()  [unwired: 4 in, 2 out]
                n310 = call "Get INI Section.vi"("Ring Refnum"=w550, "configuration file path"=w541) -> ()  [unwired: 4 in, 2 out]
                n311 = call "Get INI Section.vi"("Ring Refnum"=w551, "configuration file path"=w541) -> ()  [unwired: 4 in, 2 out]
                n312 = call "Get INI Section.vi"("Ring Refnum"=w552, "configuration file path"=w541) -> ()  [unwired: 4 in, 2 out]
                n313 = call "Get INI Section.vi"("Ring Refnum"=w553, "configuration file path"=w541) -> ()  [unwired: 4 in, 2 out]
                n314 = property on="Threat 2" class="Ring (strict)"("Strings []"=w575) -> ()  [unwired: 2 in, 2 out]
                n315 = local write "maxDev"(w571) -> ()
                n316 = local write "Impact/Target Dist"(w570) -> ()
                n317 = local write "Residual/Target Dist"(w569) -> ()
                n318 = local write "mid_to_targ_dist"(w563) -> ()
                n319 = control-ref of="Model"() -> (w542:refnum<vi>)
                n320 = control-ref of="covering"() -> (w559:refnum<vi>)
                n321 = control-ref of="shooter"() -> (w560:refnum<vi>)
                n322 = control-ref of="recorder"() -> (w561:refnum<vi>)
                n323 = control-ref of="weapon"() -> (w562:refnum<vi>)
                n324 = control-ref of="Fabric.stitch"() -> (w545:refnum<vi>)
                n325 = case shown="True" w540 {
                  tunnel: [errorcluster {"status"=FALSE, "code"=0, "source"=""} ("error out") w593] -> w568
                  tunnel: [-1 ("index of element") w591] -> w567
                  tunnel: w539 -> [_ w590]
                  tunnel: w543 -> [_ w587]
                  frame False {
                    # "Refresh"
                  }
                  frame True {
                    w589 = u8 2 ("Disabled")
                    n326 = control-ref of="projectileType"() -> (w583:refnum<vi>)
                    n327 = local read "Data Source"() -> (w592:u16)
                    n328 = call "Get Last Record (SubVI).vi"("connect Str"=w590) -> ("shot record"=→"Shot":i32, "experiment record"=w585:i32, "error out"=w593:errorcluster)
                    "Panel" <- w585
                    n329 = Build Array (concatenate)(w587, w583) -> (w586:refnum<vi>[])
                    n330 = for {
                      tunnel: w586 -> [w595] mode=indexing
                      n331 = property class="Ring (strict)"(reference=w595, "Strings []"=string[] []) -> ()  [unwired: 1 in, 2 out]
                    }
                    n332 = To Double Precision Float(number=w585) -> (double precision float=w584:dbl)
                    n333 = property on="Accept Data" class="Bool (strict)"("Disabled"=u8 0) -> ()  [unwired: 2 in, 2 out]
                    n334 = property on="Reject shot" class="Bool"("Disabled"=w589) -> ()  [unwired: 2 in, 2 out]
                    n335 = property on="Save" class="Bool"("Disabled"=w589) -> ()  [unwired: 2 in, 2 out]
                    n336 = property on="Clear" class="Bool"("Disabled"=w589) -> ()  [unwired: 2 in, 2 out]
                    n337 = case shown="2" w592 {
                      tunnel: [-1 ("index of element") -1 ("index of element") 8 ("index of element")] -> w591
                      frame 0, Default {
                      }
                      frame 1 {
                      }
                      frame 2 {
                        # "check for\nPCI 6602"
                      }
                    }
                    n338 = property on="Record #" class="DigNum (strict)"("Maximum"=w584) -> ()  [unwired: 2 in, 2 out]
                  }
                }
                n339 = call "Get INI Section.vi"("Ring Refnum"=w559, "configuration file path"=w541) -> ()  [unwired: 4 in, 2 out]
                n340 = call "Get INI Section.vi"("Ring Refnum"=w560, "configuration file path"=w541) -> ()  [unwired: 4 in, 2 out]
                n341 = call "Get INI Section.vi"("Ring Refnum"=w561, "configuration file path"=w541) -> ()  [unwired: 4 in, 2 out]
                n342 = call "Get INI Section.vi"("Ring Refnum"=w562, "configuration file path"=w541) -> ()  [unwired: 4 in, 2 out]
                n343 = call "Get INI Section.vi"("Ring Refnum"=w545, "configuration file path"=w541) -> ()  [unwired: 4 in, 2 out]
                n344 = call "Get INI Section.vi"("Ring Refnum"=w542, "configuration file path"=w541) -> ()  [unwired: 4 in, 2 out]
                n345 = Path To String(path=w541) -> (string=w572:string)
                n346 = case shown="True" "message control" {
                  tunnel: w568 -> [_ _]
                  tunnel: w572 -> [_ w579]
                  frame False {
                  }
                  frame True {
                    n347 = local write "message control"(FALSE) -> ()
                    n348 = call "Ballistics Message Center.vi"("INI File Name"=w579) -> ()
                  }
                }
                n349 = control-ref of="projectileWt"() -> (w544:refnum<vi>)
                n350 = call "Load Threats.vi"("projectileWt"=w544, "connectString"=w539) -> ()  [unwired: 1 out]
                "connStr" <- w539
              }
              frame #2 {
                n351 = One Button Dialog(message="DuBAM is now ready for use") -> ()  [unwired: 1 in, 1 out]
              }
            }
          }
        }
      }
      frame 2 {
        w664 = TRUE  # append on new line? (F)
        w704 = TRUE  # append on new line? (F)
        w736 = FALSE  # show grid lines
        w748 = -1 ("index of element")
        # "DUPONT V50 REPORT"
        # "This section prepares a DuPont V50 report (HTML)"
        # "add graph to 3rd box"
        n352 = invoke on="Shot Graph" class="XYGraph (strict)" method="Reinit To Default"() -> (error out=w717:errorcluster)  [unwired: 3 in, 2 out]
        n353 = property on="Submitter" class="Ring (strict)"() -> ("Strings []"=w651:string[], "Value"=w650:u16)  [unwired: 2 in, 2 out]
        n354 = control-ref of="Complete"() -> (w625:refnum<vi>)
        n355 = control-ref of="Points"() -> (w714:refnum<vi>)
        n356 = control-ref of="Partial"() -> (w713:refnum<vi>)
        n357 = To Long Integer(number=w650) -> (32bit integer=w624:i32)
        n358 = control-ref of="Value"() -> (w715:refnum<vi>)
        n359 = call "Graph V50.vi"("valueRef"=w715, "completeRef"=w625, "pointsRef"=w714, "partialRef"=w713, "error IN"=w717) -> ("shotGraph"=→"Shot Graph":cluster{i32[], sgl[]}[])
        n360 = Index Array(array=w651, index=w624) -> (element=w647:string)
        n361 = call <vilib>:"New Report.vi"("report type"=T11."HTML", "error in (no error)"=w717) -> ("report out"=w738:refnum<class "NI_report.lvclass">, "error out"=w737:errorcluster)  [unwired: 12 in]
        n362 = local read "Panel"() -> (w646:i32)
        n363 = Format Into String(format string="Serial Number: %5d<newline>Submitter: %s" ("Format String"), w646, w647) -> (resulting string=w645:string)  [unwired: 2 in, 1 out]
        n364 = call-dynamic "Set Report Font.vi"("report in"=w738, "text options"=T10 {"Italic"=enum."Italic Unchanged", "Strike Through"=enum."Strike Through Unchanged", "Underline"=enum."Underline Unchanged", "Bold"=enum."Bold On"}, "font settings"=T9 {"Charset (-1)"=-1, "Weight (-1)"=-1, "Name"="Arial", "Size"="4 "}, "error in (no error)"=w737) -> ("report out"=w722:refnum<class "NI_report.lvclass">, "error out"=w723:errorcluster)  [unwired: 9 in, 1 out]
        n365 = call-dynamic "Set Report Header Text.vi"("report in"=w722, "left header text"=w645, "center header text"="Ballistic V50 Report", "error in (no error)"=w723, "HTML header size"=enum16{"H1", "H2", "H3", "H4", "H5", "H6", "H7"}."H2") -> ("report out"=w725:refnum<class "NI_report.lvclass">, "error out"=w726:errorcluster)  [unwired: 9 in]
        n366 = local read "Fabric Description"() -> (w676:string)
        n367 = local read "Projectile Mass"() -> (w630:sgl)
        n368 = local read "Impact factor"() -> (w673:sgl)
        n369 = property on="Manufacturer" class="Ring (strict)"() -> ("Strings []"=w683:string[], "Value"=w682:u16)  [unwired: 2 in, 2 out]
        n370 = property on="Panel Backing" class="Ring (strict)"() -> ("Strings []"=w681:string[], "Value"=w680:u16)  [unwired: 2 in, 2 out]
        n371 = property on="Powder Type" class="Ring (strict)"() -> ("Strings []"=w679:string[], "Value"=w678:u16)  [unwired: 2 in, 2 out]
        n372 = property on="Threat 2" class="Ring (strict)"() -> ("Strings []"=w675:string[], "Value"=w674:u16)  [unwired: 2 in, 2 out]
        n373 = local read "RoomT"() -> (w632:i32)
        n374 = call-dynamic "Set Report Font.vi"("report in"=w725, "text options"=T10 {"Italic"=enum."Italic Unchanged", "Strike Through"=enum."Strike Through Unchanged", "Underline"=enum."Underline Unchanged", "Bold"=enum."Bold Off"}, "font settings"=T9 {"Charset (-1)"=-1, "Weight (-1)"=-1, "Name"="Arial", "Size"="1"}, "error in (no error)"=w726) -> ("report out"=w701:refnum<class "NI_report.lvclass">, "error out"=w702:errorcluster)  [unwired: 9 in, 1 out]
        n375 = Select(t="Disclosure on Ballistic and Stab Test Data<newline>The attached ballistic test data was generated by DuPont and corresponds to DuPont's current knowledge on the performance of the subject test panels against certain ballistic threats.  This information is offered solely to provide possible suggestions for your own experimentation and validation.  It is not intended as a substitute for your own testing or any testing you may need to submit for a bid package, you should undertake your own testing whether you do so yourself with the supplier of the materials to be tested or with an independent, third party, certified testing facility and the supplier of the materials to be tested (i.e., the fabric weaver).  DuPont makes no warranties, and assumes no liabilities in connection with any use of the information supplied with this disclosure statement." ("text"), s="Add Disclaimer", f="" ("t")) -> (s? t:f=w660:string)
        n376 = To Long Integer(number=w682) -> (32bit integer=w613:i32)
        n377 = To Long Integer(number=w680) -> (32bit integer=w616:i32)
        n378 = To Long Integer(number=w678) -> (32bit integer=w615:i32)
        n379 = To Long Integer(number=w674) -> (32bit integer=w614:i32)
        n380 = Index Array(array=w683, index=w613) -> (element=w677:string)
        n381 = call-poly <vilib>:"Append Report Text.vi"("report in"=w701, "text"=w660, "error in (no error)"=w702) -> ("report out"=w700:refnum<class "NI_report.lvclass">, "error out"=w698:errorcluster)  [unwired: 9 in, 2 out]
        n382 = Index Array(array=w681, index=w616) -> (element=w629:string)
        n383 = Index Array(array=w679, index=w615) -> (element=w667:string)
        n384 = Index Array(array=w675, index=w614) -> (element=w635:string)
        n385 = property on="Test Conditions" class="Ring (strict)"() -> ("Strings []"=w672:string[], "Value"=w671:u16)  [unwired: 2 in, 2 out]
        n386 = property on="Panel Type" class="Ring (strict)"() -> ("Strings []"=w670:string[], "Value"=w669:u16)  [unwired: 2 in, 2 out]
        n387 = local read "Z.M.R."() -> (w658:sgl)
        n388 = call-dynamic "Set Report Font.vi"("report in"=w700, "text options"=T10 {"Italic"=enum."Italic Unchanged", "Strike Through"=enum."Strike Through Unchanged", "Underline"=enum."Underline Unchanged", "Bold"=enum."Bold Unchanged"}, "font settings"=T9 {"Charset (-1)"=-1, "Weight (-1)"=-1, "Name"="Arial", "Size"="3 "}, "error in (no error)"=w698) -> ("report out"=w699:refnum<class "NI_report.lvclass">, "error out"=w697:errorcluster)  [unwired: 9 in, 1 out]
        n389 = local read "Weight of Panel"() -> (w631:dbl)
        n390 = local read "Areal Density"() -> (w628:dbl)
        n391 = local read "Sample #"() -> (w627:string)
        n392 = local read "Shot Angle"() -> (w666:u16)
        n393 = local read "RoomHum"() -> (w634:i32)
        n394 = call-dynamic "New Report Line.vi"("report in"=w699, "error in (no error)"=w697) -> ("report out"=w739:refnum<class "NI_report.lvclass">, "error out"=w740:errorcluster)  [unwired: 12 in]
        n395 = To Long Integer(number=w671) -> (32bit integer=w612:i32)
        n396 = To Long Integer(number=w669) -> (32bit integer=w611:i32)
        n397 = Index Array(array=w672, index=w612) -> (element=w665:string)
        n398 = call-dynamic "New Report Line.vi"("report in"=w739, "error in (no error)"=w740) -> ("report out"=w706:refnum<class "NI_report.lvclass">, "error out"=w705:errorcluster)  [unwired: 12 in]
        n399 = Index Array(array=w670, index=w611) -> (element=w633:string)
        n400 = Format Into String(format string="<table border=\"0\" cellspacing=\"6\"><tr><td align=\"left\"><b>Fabric Parameters</b></td><td>&nbsp;</td><td>&nbsp;</td><td align=\"left\"><b>Test Parameters</b></td><td>&nbsp;</td></tr><tr><td align=\"right\">Sample ID: </td><td align=\"left\">%s</td><td>&nbsp;</td><td align=\"right\">Method: </td><td align=\"left\">V50</td></tr><tr><td align=\"right\">Areal Density: </td><td align=\"left\">%.3f</td><td>&nbsp;</td><td align=\"right\">Threat: </td><td align=\"left\">%s</td></tr><tr><td align=\"right\">Manufacturer: </td><td align=\"left\">%s</td><td>&nbsp;</td><td align=\"right\">Room Temperature: </td><td align=\"left\">%.0f</td></tr><tr><td align=\"right\">Group Data: </td><td align=\"left\">%s</td><td>&nbsp;</td><td align=\"right\">Correction Factor: </td><td align=\"left\">%0.4f</td></tr><tr><td align=\"right\">Projectile Weight: </td><td align=\"left\">%0.3f</td><td>&nbsp;</td><td align=\"right\">Panel Backing: </td><td align=\"left\">%s</td></tr><tr><td align=\"right\">Powder Type: </td><td align=\"left\">%s</td><td>&nbsp;</td><td align=\"right\">Shot Angle: </td><td align=\"left\">%.0f</td></tr><tr><td align=\"right\">Test Conditions: </td><td align=\"left\">%s</td><td>&nbsp;</td><td align=\"right\">Room Humidity: </td><td align=\"left\">%.0f</td></tr><tr><td align=\"right\">Panel Weight: </td><td align=\"left\">%.4f</td><td>&nbsp;</td><td>&nbsp;</td></tr><tr><td align=\"right\">Descripton: </td><td align=\"left\">%s</td><td>&nbsp;</td><td>&nbsp;</td></tr></table>", w627, w628, w635, w677, w632, w676, w673, w630, w629, w667, w666, w665, w634, w631, w633) -> (resulting string=w662:string)  [unwired: 2 in, 1 out]
        n401 = property on="ballistician" class="Ring (strict)"() -> ("Strings []"=w687:string[], "Value"=w686:u16)  [unwired: 2 in, 2 out]
        n402 = call-poly <vilib>:"Append Report Text.vi"("report in"=w706, "text"=w662, "append on new line? (F)"=w704, "error in (no error)"=w705) -> ("report out"=w639:refnum<class "NI_report.lvclass">, "error out"=w640:errorcluster)  [unwired: 8 in, 2 out]
        n403 = To Long Integer(number=w686) -> (32bit integer=w610:i32)
        n404 = call-dynamic "New Report Line.vi"("report in"=w639, "error in (no error)"=w640) -> ("report out"=w733:refnum<class "NI_report.lvclass">, "error out"=w734:errorcluster)  [unwired: 12 in]
        n405 = local read "computed_V50"() -> (w703:sgl)
        n406 = Get Date/Time String(date format (0)=enum16{"short", "long", "abbreviated"}."abbreviated") -> (date string=w694:string)  [unwired: 2 in, 1 out]
        n407 = Index Array(array=w687, index=w610) -> (element=w685:string)
        n408 = local read "Sample #"() -> (w649:string)
        n409 = property on="Table of Shots" class="Tbl (strict)"() -> ("Column Header Strings[]"=w716:string[])  [unwired: 2 in, 2 out]
        n410 = Less Than 0?(x=w658) -> (x < 0?=w659:bool)
        n411 = call-dynamic "New Report Line.vi"("report in"=w733, "error in (no error)"=w734) -> ("report out"=w732:refnum<class "NI_report.lvclass">, "error out"=w731:errorcluster)  [unwired: 12 in]
        n412 = Concatenate Strings(w694, " © " ("right footer text"), "  DuPont ") -> (w710:string)
        n413 = local read "Pairs"() -> (w684:i16)
        n414 = Select(t="Low Complete-High Partial: ", s=w659, f="Zone of Mixed Results: ") -> (s? t:f=w654:string)
        n415 = Format Value(format string="Panel %s.html  " ("string (\"\")"), value (0)=w649) -> (output string=w709:string)  [unwired: 1 in]
        n416 = call-poly <vilib>:"Append Table to Report.vi"("report in"=w732, "column width (1)"=1.1, "column headers"=w716, "text data"="Table of Shots", "error in (no error)"=w731, "show grid lines"=w736) -> ("report out"=w688:refnum<class "NI_report.lvclass">, "error out"=w692:errorcluster)  [unwired: 6 in, 2 out]
        n417 = Build Path(base path="Report Path", name or relative path=w709) -> (appended path=w707:path)
        n418 = Concatenate Strings(" V50:  %10.1f<newline>Number of Pairs Used: %d<newline>  ", w654, "%.1f<newline><newline>Ballistician:%s<newline> ") -> (w652:string)
        n419 = Format Into String(format string=w652, w703, w684, w658, w685) -> (resulting string=w623:string)  [unwired: 2 in, 1 out]
        n420 = call-dynamic "Set Report Font.vi"("report in"=w688, "text options"=T10 {"Italic"=enum."Italic Unchanged", "Strike Through"=enum."Strike Through Unchanged", "Underline"=enum."Underline On", "Bold"=enum."Bold Off"}, "font settings"=T9 {"Charset (-1)"=-1, "Weight (-1)"=-1, "Name"="Arial", "Size"="3 "}, "error in (no error)"=w692) -> ("report out"=w689:refnum<class "NI_report.lvclass">, "error out"=w690:errorcluster)  [unwired: 9 in, 1 out]
        n421 = call-dynamic "New Report Line.vi"("report in"=w689, "error in (no error)"=w690) -> ("report out"=w730:refnum<class "NI_report.lvclass">, "error out"=w729:errorcluster)  [unwired: 12 in]
        n422 = control-ref of="Shot Graph"() -> (w663:refnum<vi>)
        n423 = call-poly <vilib>:"Append Report Text.vi"("report in"=w730, "text"=w623, "append on new line? (F)"=w664, "error in (no error)"=w729) -> ("report out"=w637:refnum<class "NI_report.lvclass">, "error out"=w636:errorcluster)  [unwired: 8 in, 2 out]
        n424 = call-dynamic "Append Control Image to Report.vi"("report in"=w637, "image file type (.jpg)"=enum16{".jpg", ".png"}.".jpg" ("image file type(.png)"), "ctrl reference"=w663, "description"="Graph of Test Results" ("control name"), "error in (no error)"=w636) -> ("report out"=w622:refnum<class "NI_report.lvclass">, "error out"=w621:errorcluster)  [unwired: 7 in, 2 out]
        n425 = call-dynamic "Set Report Footer Text.vi"("report in"=w622, "right footer text"=w710, "error in (no error)"=w621) -> ("report out"=w727:refnum<class "NI_report.lvclass">, "error out"=w728:errorcluster)  [unwired: 11 in]
        n426 = call-dynamic "Get Report Type.vi"("report in"=w727, "error in (no error)"=w728) -> ("report out"=w744:refnum<class "NI_report.lvclass">, "report type"=w743:T11, "error out"=w747:errorcluster)  [unwired: 11 in]
        n427 = case shown="\"Standard Report\", Default" w743 {
          tunnel: w744 -> [w753 w758 w760 w762]
          tunnel: [w752 w757 w760 w762] -> w745
          tunnel: [w751 w756 w759 w761] -> w746
          tunnel: w747 -> [w750 w755 w759 w761]
          tunnel: w707 -> [_ w754 _ _]
          frame "Standard Report", Default {
            n428 = call-dynamic "Print Report.vi"("report in"=w753, "error in (no error)"=w750) -> ("report out"=w752:refnum<class "NI_report.lvclass">, "error out"=w751:errorcluster)  [unwired: 12 in]
          }
          frame "HTML" {
            n429 = call-dynamic "Save Report to File.vi"("report in"=w758, "report file path"=w754, "error in (no error)"=w755) -> ("report out"=w757:refnum<class "NI_report.lvclass">, "error out"=w756:errorcluster)  [unwired: 11 in]
          }
          frame "Word" {
          }
          frame "Excel" {
          }
        }
        n430 = call-dynamic "Dispose Report.vi"("report in"=w745, "error in (no error)"=w746) -> ("error out"=w641:errorcluster)  [unwired: 13 in]
        n431 = call <vilib>:"Simple Error Handler.vi"("error in (no error)"=w641) -> ("error out"=w642:errorcluster)  [unwired: 4 in, 4 out]
        n432 = case shown="No Error" w642 {
          frame No Error {
            n433 = One Button Dialog(message="A V50 Report is ready.") -> ()  [unwired: 1 in, 1 out]
          }
          frame Error {
          }
        }
      }
      frame 3 {
        w797 = TRUE  # Enable
        w800 = -1 ("index of element")
        # "DHB BALLISTIC TEST REPORT"
        # "The custom Excel template file is \nexpected in the C:\\Ballistics folder."
        # "Create DHB Ballistic Test Report"
        n434 = case shown="True" "lookupRec" {
          selector: "lookupRec" -> [_ w1082]
          tunnel: [w818 w1061] -> w795
          tunnel: [w817 w1045] -> w794
          tunnel: [w816 w1065] -> w793
          tunnel: [w815 w1070] -> w792
          tunnel: [w814 w1063] -> w791
          tunnel: [w813 w1067] -> w790
          tunnel: w776 -> [w812 _]
          tunnel: w775 -> [w811 _]
          tunnel: w774 -> [w810 _]
          tunnel: w773 -> [w809 _]
          tunnel: [w808 w1073] -> w772
          tunnel: [w807 w1077] -> w771
          tunnel: [w806 w1076] -> w770
          tunnel: [w805 "Record #"] -> w769
          tunnel: [w804 w1064] -> w768
          tunnel: [w803 w1075] -> w767
          tunnel: w764 -> [_ w1062]
          tunnel: w763 -> [w802 _]
          frame False {
            n435 = stacked-sequence {
              tunnel: [_ _ _ _ _ w1005 _] -> w813
              tunnel: [_ w880 _ _ _ _ _] -> w817
              tunnel: [_ _ _ _ w964 _ _] -> w814
              tunnel: [_ _ _ w930 _ _ _] -> w815
              tunnel: [_ _ w902 _ _ _ _] -> w816
              tunnel: [w823 _ _ _ _ _ _] -> w818
              tunnel: w811 -> [w822 _ _ _ _ _ _]
              tunnel: w812 -> [w821 _ _ _ _ _ _]
              tunnel: w810 -> [w820 _ _ _ _ _ _]
              tunnel: w809 -> [w819 _ _ _ _ _ _]
              tunnel: [_ _ _ _ _ _ w1030] -> w808
              tunnel: [_ _ _ _ _ _ w1029] -> w807
              tunnel: [_ _ _ _ _ _ w1028] -> w806
              tunnel: [_ _ _ _ _ _ w1027] -> w805
              tunnel: [_ _ _ _ _ _ w1026] -> w804
              tunnel: [_ _ _ _ _ _ w1025] -> w803
              tunnel: w802 -> [_ _ w901 _ w957 _ _]
              tunnel: "Method" -> [_ _ w892 _ w956 _ _]
              frame #0 {
                # "FABRIC"
                n436 = local read "fab1_totalWt"() -> (w826:sgl)
                n437 = local read "fab3_totalWt"() -> (w828:sgl)
                n438 = local read "fab5_totalWt"() -> (w830:sgl)
                n439 = local read "fab2_totalWt"() -> (w827:sgl)
                n440 = local read "fab4_totalWt"() -> (w829:sgl)
                n441 = local read "fab6_totalWt"() -> (w831:sgl)
                n442 = Build Array(w826, w827, w828, w829, w830, w831) -> (w825:sgl[])
                n443 = for {
                  tunnel: w825 -> [w832] mode=indexing
                  tunnel: [w839] -> w824 mode=indexing
                  tunnel: w821 -> [w837] mode=indexing
                  tunnel: w822 -> [w836] mode=indexing
                  tunnel: w820 -> [w835] mode=indexing
                  tunnel: w819 -> [w834] mode=indexing
                  n444 = Unbundle By Name(w836) -> ("plyNum"=w833:i32)
                  n445 = Less Or Equal To 0?(x=w832) -> (x <= 0?=w838:bool)
                  n446 = case shown="False" w838 {
                    tunnel: [w863 w865] -> w839
                    tunnel: w832 -> [w862 _]
                    tunnel: w837 -> [w858 _]
                    tunnel: w836 -> [w857 _]
                    tunnel: w835 -> [w850 _]
                    tunnel: w834 -> [w847 _]
                    tunnel: w833 -> [w843 _]
                    frame False {
                      n447 = Unbundle By Name(w858) -> ("fabricID_DHB"=w844:string, "Fabric.fiber"=w845:string, "Fabric.denier"=w852:string, "pick"=w851:string, "weave"=w840:string, "finish"=w841:string, "ozPerYd2"=w855:string)
                      n448 = Unbundle By Name(w857) -> ("LotNum"=w853:string, "RollNum"=w854:string, "Fabric.stitch"=w856:u16)
                      n449 = Format Into String(w843) -> (resulting string=w849:string)  [unwired: 3 in, 1 out]
                      n450 = To Long Integer(number=w856) -> (32bit integer=w861:i32)
                      n451 = call "Dropdown Selection (SubVI).vi"("reference"=w850) -> ("element"=w848:string)
                      n452 = call "Dropdown Selection (SubVI).vi"("reference"=w847) -> ("element"=w846:string)
                      n453 = property on="Fabric.stitch" class="Ring (strict)"() -> ("Strings []"=w842:string[])  [unwired: 2 in, 2 out]
                      n454 = Index Array(array=w842, index=w861) -> (element=w859:string)
                      n455 = Format Into String(w862) -> (resulting string=w860:string)  [unwired: 3 in, 1 out]
                      n456 = Build Array(w849, w848, w846, w844, w845, w852, w851, w840, w841, w853, w854, w855, w860, w859) -> (w863:string[])
                    }
                    frame True {
                      n457 = call <vilib>:"Space Constant.vi"() -> ("String"=w866:string)
                      n458 = Initialize Array(w866, 12 ("dimension size")) -> (w865:string[])
                    }
                  }
                }
                n459 = Transpose 2D Array(2D array=w824) -> (transposed array=w823:string[][])
              }
              frame #1 {
                # "muzzel / midpoint"
                # "muzzle / scr#1"
                # "muzzle / target"
                # "scr#2 / target"
                # "RANGE"
                n460 = local read "Impact/Separation"() -> (w873:sgl)
                n461 = local read "mid_to_targ_dist"() -> (w870:sgl)
                n462 = local read "Barrel to Screen"() -> (w867:sgl)
                n463 = local read "clayAverage"() -> (w889:sgl)
                n464 = Divide(x=w873, y=sgl 2.0) -> (x/y=w868:sgl)
                n465 = local read "RoomHum"() -> (w884:i32)
                n466 = local read "clayTemp"() -> (w887:i16)
                n467 = local read "clayCalib"() -> (w890:string)
                n468 = local read "RoomT"() -> (w885:i32)
                n469 = Add(x=w867, y=w870) -> (x+y=w874:sgl)
                n470 = Subtract(x=w867, y=w868) -> (x-y=w869:sgl)
                n471 = Subtract(x=w870, y=w868) -> (x-y=w871:sgl)
                n472 = Format Into String(w874) -> (resulting string=w875:string)  [unwired: 3 in, 1 out]
                n473 = Format Into String(w869) -> (resulting string=w876:string)  [unwired: 3 in, 1 out]
                n474 = Format Into String(w873) -> (resulting string=w877:string)  [unwired: 3 in, 1 out]
                n475 = Format Into String(w871) -> (resulting string=w878:string)  [unwired: 3 in, 1 out]
                n476 = Format Into String(w870) -> (resulting string=w879:string)  [unwired: 3 in, 1 out]
                n477 = Format Into String(w884) -> (resulting string=w882:string)  [unwired: 3 in, 1 out]
                n478 = Format Into String(w885) -> (resulting string=w883:string)  [unwired: 3 in, 1 out]
                n479 = Format Into String(format string="%d", w887) -> (resulting string=w886:string)  [unwired: 2 in, 1 out]
                n480 = Format Into String(w889) -> (resulting string=w888:string)  [unwired: 3 in, 1 out]
                n481 = Bundle(w875, w876, w877, w878, w879, w882, w883, w886, "clayCalib"=w890, w888) -> (w891:T15)  [unwired: 1 in]
                n482 = Cluster To Array(cluster=w891) -> (array=w880:string[])
              }
              frame #2 {
                # "RESULTS"
                n483 = for {
                  tunnel: w901 -> [w929] mode=indexing
                  tunnel: [w928] -> w900 mode=indexing
                  tunnel: [w927] -> w899
                  i -> [w927]
                  n484 = Unbundle By Name(w929) -> ("BackFace\nDepth"=w928:sgl)
                }
                n485 = Increment(x=w899) -> (x+1=w897:i32)
                n486 = Add Array Elements(numeric array=w900) -> (sum=w898:sgl)
                n487 = To Single Precision Float(number=w897) -> (single precision float=w896:sgl)
                n488 = Divide(x=w898, y=w896) -> (x/y=w895:sgl)
                n489 = Format Into String(format string="%1.1f", w895) -> (resulting string=w894:string)  [unwired: 2 in, 1 out]
                n490 = case shown="1, 2" w892 {
                  tunnel: [w917 w926] -> w904
                  tunnel: w894 -> [w905 w925]
                  frame 0, Default {
                    w911 = "%1d" ("format string")
                    n491 = local read "Z.M.R."() -> (w909:sgl)
                    n492 = Less Than 0?(x=w909) -> (x < 0?=w910:bool)
                    n493 = local read "rangeOfResults"() -> (w913:i32)
                    n494 = local read "computed_V50"() -> (w916:sgl)
                    n495 = local read "lowComplete"() -> (w914:i32)
                    n496 = local read "highPartial"() -> (w915:i32)
                    n497 = case shown="True" w910 {
                      tunnel: w909 -> [w922 _]
                      tunnel: [w922 sgl 0.0 ("Z.M.R.")] -> w908
                      frame False {
                      }
                      frame True {
                      }
                    }
                    n498 = Format Into String(format string="%1.1f", w916) -> (resulting string=w920:string)  [unwired: 2 in, 1 out]
                    n499 = Format Into String(format string=w911, w915) -> (resulting string=w919:string)  [unwired: 2 in, 1 out]
                    n500 = Format Into String(format string=w911, w914) -> (resulting string=w918:string)  [unwired: 2 in, 1 out]
                    n501 = Format Into String(format string=w911, w913) -> (resulting string=w921:string)  [unwired: 2 in, 1 out]
                    n502 = Format Into String(format string="%1.1f", w908) -> (resulting string=w907:string)  [unwired: 2 in, 1 out]
                    n503 = Bundle(w920, w919, w918, w921, w907, w905, w905) -> (w917:T16)  [unwired: 1 in]
                  }
                  frame 1, 2 {
                    w924 = ""
                    n504 = Bundle(w924, w924, w924, w924, w924, w925, w925) -> (w926:T16)  [unwired: 1 in]
                  }
                }
                n505 = Cluster To Array(cluster=w904) -> (array=w903:string[])
                n506 = Build Array(w903) -> (w902:string[][])
              }
              frame #3 {
                # "SAMPLE"
                n507 = control-ref of="Method"() -> (w931:refnum<vi>)
                n508 = call "Dropdown Selection (SubVI).vi"("reference"=w931) -> ("element"=w933:string)
                n509 = Equal?(x=w933, y="V50") -> (x = y?=w932:bool)
                n510 = local read "totalSampleWt"() -> (w943:sgl)
                n511 = case shown="True" w932 {
                  tunnel: ["n/a" w955] -> w937
                  frame False {
                  }
                  frame True {
                    n512 = local read "minV50"() -> (w954:i32)
                    n513 = Format Into String(w954) -> (resulting string=w955:string)  [unwired: 3 in, 1 out]
                  }
                }
                n514 = control-ref of="Panel Dimensions"() -> (w950:refnum<vi>)
                n515 = control-ref of="workType"() -> (w951:refnum<vi>)
                n516 = control-ref of="covering"() -> (w952:refnum<vi>)
                n517 = control-ref of="Model"() -> (w936:refnum<vi>)
                n518 = local read "serialNum"() -> (w945:string)
                n519 = local read "Thickness"() -> (w940:dbl)
                n520 = local read "Sample #"() -> (w948:string)
                n521 = local read "totalBAW"() -> (w939:sgl)
                n522 = call "Dropdown Selection (SubVI).vi"("reference"=w950) -> ("element"=w947:string)
                n523 = call "Dropdown Selection (SubVI).vi"("reference"=w951) -> ("element"=w946:string)
                n524 = call "Dropdown Selection (SubVI).vi"("reference"=w936) -> ("element"=w935:string)
                n525 = call "Dropdown Selection (SubVI).vi"("reference"=w952) -> ("element"=w944:string)
                n526 = Format Into String(w943) -> (resulting string=w942:string)  [unwired: 3 in, 1 out]
                n527 = Format Into String(w940) -> (resulting string=w941:string)  [unwired: 3 in, 1 out]
                n528 = Format Into String(w939) -> (resulting string=w938:string)  [unwired: 3 in, 1 out]
                n529 = Bundle("Sample #"=w948, "element"=w947, "element"=w946, "serialNum"=w945, "element"=w935, w942, w941, w938, "element"=w944, w937) -> (w949:T17)  [unwired: 1 in]
                n530 = Cluster To Array(cluster=w949) -> (array=w930:string[])
              }
              frame #4 {
                # "SHOT TABLE"
                n531 = for {
                  tunnel: w957 -> [w996] mode=indexing
                  shift-right: [w973] -> _
                  shift-left: T12 [] -> [w975]
                  tunnel: [w973] -> w960
                  tunnel: w956 -> [w969]
                  n532 = Unbundle By Name(w996) -> ("shot order"=w995:i32, "Powder Loading"=w994:sgl, "Uncorrected Impact"=w993:sgl, "UncorrectedRed_PB"=w992:sgl, "UncorrectedAvgVel_PB"=w991:sgl, "velLoss_PB"=w990:sgl, "strikeVel_PB"=w989:sgl, "SHOT STATUS"=w978:u16, "usedv50"=w988:bool, "Shot Angle"=w970:u16, "BackFace\nDepth"=w971:sgl)
                  n533 = case shown="0, Default" w969 {
                    tunnel: w988 -> [w998 _]
                    tunnel: [w997 w1002] -> w987
                    tunnel: w970 -> [_ w1001]
                    frame 0, Default {
                      n534 = case shown="True" w998 {
                        tunnel: ["" ("Empty String Constant") "*"] -> w997
                        frame False {
                        }
                        frame True {
                        }
                      }
                    }
                    frame 1, 2 {
                      n535 = Format Into String(w1001) -> (resulting string=w1002:string)  [unwired: 3 in, 1 out]
                    }
                  }
                  n536 = case shown="1" w978 {
                    tunnel: ["P" "C"] -> w977
                    frame 0, Default {
                    }
                    frame 1 {
                    }
                  }
                  n537 = Format Into String(format string="%2d", w995) -> (resulting string=w980:string)  [unwired: 2 in, 1 out]
                  n538 = Format Into String(w994) -> (resulting string=w981:string)  [unwired: 3 in, 1 out]
                  n539 = Format Into String(w993) -> (resulting string=w982:string)  [unwired: 3 in, 1 out]
                  n540 = Format Into String(w992) -> (resulting string=w983:string)  [unwired: 3 in, 1 out]
                  n541 = Format Into String(w991) -> (resulting string=w984:string)  [unwired: 3 in, 1 out]
                  n542 = Format Into String(w990) -> (resulting string=w985:string)  [unwired: 3 in, 1 out]
                  n543 = Format Into String(w989) -> (resulting string=w986:string)  [unwired: 3 in, 1 out]
                  n544 = Format Into String(w971) -> (resulting string=w979:string)  [unwired: 3 in, 1 out]
                  n545 = Build Array(w980, w981, w982, w983, w984, w985, w986, w977, w987, w979) -> (w974:string[])
                  n546 = Array To Cluster(array=w974) -> (cluster=w976:T18)
                  n547 = Build Array (concatenate)(w975, w976) -> (w973:T12)
                }
                n548 = Array Size(array=w960) -> (size(s)=w962:i32)
                n549 = Equal To 0?(x=w962) -> (x = 0?=w958:bool)
                n550 = case shown="True" w958 {
                  tunnel: [w965 T12 [{"[0]"="", "[1]"="", "[2]"="", "[3]"="", "[4]"="", "[5]"="", "[6]"="", "[7]"="", "[8]"="", "[9]"=""}]] -> w959
                  tunnel: w960 -> [w965 _]
                  frame False {
                  }
                  frame True {
                  }
                }
                n551 = Sort 1D Array(array=w959) -> (sorted array=w961:T12)
                n552 = for {
                  tunnel: w961 -> [w968] mode=indexing
                  tunnel: [w967] -> w964 mode=indexing
                  n553 = Cluster To Array(cluster=w968) -> (array=w967:string[])
                }
              }
              frame #5 {
                # "THREAT"
                n554 = local read "threatDetails"() -> (w1009:T2)
                n555 = Unbundle By Name(w1009) -> ("barrelLength"=w1008:string)
                n556 = local read "Shot Angle"() -> (w1010:u16)
                n557 = control-ref of="weapon"() -> (w1021:refnum<vi>)
                n558 = control-ref of="projectileType"() -> (w1020:refnum<vi>)
                n559 = control-ref of="projectileWt"() -> (w1006:refnum<vi>)
                n560 = control-ref of="Powder Type"() -> (w1019:refnum<vi>)
                n561 = control-ref of="rangeNum"() -> (w1022:refnum<vi>)
                n562 = control-ref of="shooter"() -> (w1024:refnum<vi>)
                n563 = control-ref of="recorder"() -> (w1023:refnum<vi>)
                n564 = Format Into String(w1010) -> (resulting string=w1011:string)  [unwired: 3 in, 1 out]
                n565 = call "Dropdown Selection (SubVI).vi"("reference"=w1021) -> ("element"=w1017:string)
                n566 = call "Dropdown Selection (SubVI).vi"("reference"=w1020) -> ("element"=w1016:string)
                n567 = call "Dropdown Selection (SubVI).vi"("reference"=w1006) -> ("element"=w1007:string)
                n568 = call "Dropdown Selection (SubVI).vi"("reference"=w1019) -> ("element"=w1015:string)
                n569 = call "Dropdown Selection (SubVI).vi"("reference"=w1022) -> ("element"=w1014:string)
                n570 = call "Dropdown Selection (SubVI).vi"("reference"=w1024) -> ("element"=w1013:string)
                n571 = call "Dropdown Selection (SubVI).vi"("reference"=w1023) -> ("element"=w1012:string)
                n572 = Bundle("element"=w1017, "element"=w1016, "element"=w1007, "element"=w1015, "barrelLength"=w1008, w1011, "element"=w1014, "element"=w1013, "element"=w1012) -> (w1018:T19)  [unwired: 1 in]
                n573 = Cluster To Array(cluster=w1018) -> (array=w1005:string[])
              }
              frame #6 {
                # "GENERAL"
                n574 = control-ref of="Method"() -> (w1031:refnum<vi>)
                n575 = control-ref of="standard"() -> (w1032:refnum<vi>)
                n576 = local read "Comments"() -> (w1026:string)
                n577 = local read "projName"() -> (w1029:string)
                n578 = local read "projNum"() -> (w1028:string)
                n579 = local read "Panel"() -> (w1033:i32)
                n580 = call "Dropdown Selection (SubVI).vi"("reference"=w1031) -> ("element"=w1030:string)
                n581 = call "Dropdown Selection (SubVI).vi"("reference"=w1032) -> ("element"=w1025:string)
                n582 = Increment(x=w1033) -> (x+1=w1027:i32)
              }
            }
          }
          frame True {
            # "method"
            # "general"
            # "remark"
            # "threat"
            # "shots"
            # "sample"
            # "results"
            # "range"
            # "fabric"
            # "query db with the entered record number and use result to populate the xlt"
            n583 = Not(x=w1082) -> (.not. x?=w1081:bool)
            n584 = local write "lookupRec"(w1081) -> ()
            n585 = Format Into String(format string="SELECT * FROM Experiment\nWHERE expt=%d;" ("query string"), "Record #") -> (resulting string=w1078:string)  [unwired: 2 in, 1 out]
            n586 = call "Fetch Data (SubVI).vi"("connectString"=w1062, "query string"=w1078) -> ("recordset data"=w1080:string[][])  [unwired: 1 in, 1 out]
            n587 = Index Array(array=w1080) -> (element=w1038:string[])  [unwired: 2 in]
            n588 = Index Array(array=w1038, index=4) -> (element=w1035:string)
            n589 = local read "Impact/Separation"() -> (w1052:sgl)
            n590 = call "Load Shots (SubVI).vi"("connectString"=w1062, "Record #"="Record #", "Method"=w1035) -> ("Shot Array"=w1063:string[][], "avgDef"=w1041:dbl)
            n591 = local read "mid_to_targ_dist"() -> (w1055:sgl)
            n592 = local read "Barrel to Screen"() -> (w1058:sgl)
            n593 = Format Into String(w1041) -> (resulting string=w1039:string)  [unwired: 3 in, 1 out]
            n594 = Match Pattern(string=w1035, regular expression="N.I.J.") -> (offset past match=w1037:i32)  [unwired: 1 in, 3 out]
            n595 = Greater Or Equal To 0?(x=w1037) -> (x >= 0?=w1034:bool)
            n596 = Divide(x=w1052, y=sgl 2.0) -> (x/y=w1057:sgl)
            n597 = case shown="True" w1034 {
              tunnel: [w1085 w1089] -> w1040
              tunnel: w1039 -> [w1084 w1091]
              tunnel: w1038 -> [w1083 _]
              frame False {
                n598 = Array Subset(array=w1083, index=141, length=5) -> (w1086:string[])
                n599 = Build Array (concatenate)(w1086, w1084, w1084) -> (w1085:string[])
              }
              frame True {
                w1090 = ""
                n600 = Build Array(w1090, w1090, w1090, w1090, w1090, w1091, w1091) -> (w1089:string[])
              }
            }
            n601 = Add(x=w1058, y=w1055) -> (x+y=w1051:sgl)
            n602 = Subtract(x=w1058, y=w1057) -> (x-y=w1056:sgl)
            n603 = Subtract(x=w1055, y=w1057) -> (x-y=w1054:sgl)
            n604 = Array Subset(array=w1038, index=33, length=5) -> (w1044:string[])
            n605 = Format Into String(w1051) -> (resulting string=w1050:string)  [unwired: 3 in, 1 out]
            n606 = Format Into String(w1056) -> (resulting string=w1049:string)  [unwired: 3 in, 1 out]
            n607 = Format Into String(w1052) -> (resulting string=w1048:string)  [unwired: 3 in, 1 out]
            n608 = Format Into String(w1054) -> (resulting string=w1047:string)  [unwired: 3 in, 1 out]
            n609 = Format Into String(w1055) -> (resulting string=w1046:string)  [unwired: 3 in, 1 out]
            n610 = Array Subset(array=w1038, index=9, length=10) -> (w1070:string[])
            n611 = Build Array (concatenate)(w1050, w1049, w1048, w1047, w1046, w1044) -> (w1045:string[])
            n612 = Array Subset(array=w1038, index=19, length=9) -> (w1067:string[])
            n613 = Index Array(array=w1038, index #1=4 ("index")) -> (element #1=w1073:string, element #2=w1075:string, element #3=w1077:string, element #4=w1076:string)  [unwired: 3 in]
            n614 = Index Array(array=w1038, index=146) -> (element=w1064:string)
            n615 = Build Array(w1040) -> (w1065:string[][])
            n616 = call "Get Model Construction.vi"("panel record"=w1038) -> ("Fabric Array"=w1061:string[][])
          }
        }
        n617 = To Variant(anything=w795) -> (Variant=w789:variant)
        n618 = To Variant(anything=w794) -> (Variant=w788:variant)
        n619 = To Variant(anything=w793) -> (Variant=w787:variant)
        n620 = To Variant(anything=w792) -> (Variant=w786:variant)
        n621 = To Variant(anything=w791) -> (Variant=w785:variant)
        n622 = To Variant(anything=w790) -> (Variant=w784:variant)
        n623 = To Variant(anything=w772) -> (Variant=w783:variant)
        n624 = To Variant(anything=w771) -> (Variant=w782:variant)
        n625 = To Variant(anything=w770) -> (Variant=w781:variant)
        n626 = To Variant(anything=w769) -> (Variant=w778:variant)
        n627 = To Variant(anything=w768) -> (Variant=w779:variant)
        n628 = To Variant(anything=w767) -> (Variant=w780:variant)
        n629 = call "MS Office Report2"("Enable"=w797, "blockFabric"=w789, "blockRange"=w788, "blockResults"=w787, "blockSample"=w786, "blockShotTbl"=w785, "blockThreat"=w784, "method"=w783, "projName"=w782, "projNum"=w781, "recNum"=w778, "remark"=w779, "standard"=w780) -> ("error out"=w796:errorcluster)  [unwired: 14 in]
        n630 = call <vilib>:"Simple Error Handler.vi"("error in (no error)"=w796) -> ("error out"=w798:errorcluster)  [unwired: 4 in, 4 out]
        n631 = case shown="No Error" w798 {
          frame No Error {
            n632 = One Button Dialog(message="A Ballistic Test  Report is ready.") -> ()  [unwired: 1 in, 1 out]
          }
          frame Error {
          }
        }
      }
      frame 4 {
        # "SAVE SHOTS"
        # "This section saves the shots to the data base"
        n633 = stacked-sequence {
          seq-local: [w1113 _ _] -> [_ w1284 _]
          seq-local: [w1112 _ _] -> [_ w1278 _]
          seq-local: [_ w1264 _] -> [_ _ w1303]
          seq-local: [_ w1266 _] -> [_ _ w1302]
          seq-local: [_ w1262 _] -> [_ _ w1295]
          seq-local: [w1122 _ _] -> [_ w1261 _]
          seq-local: [w1121 _ _] -> [_ w1260 _]
          tunnel: [_ _ w1297] -> w1101
          tunnel: [_ _ w1300] -> w1103
          tunnel: w1099 -> [w1108 _ _]
          tunnel: w1098 -> [w1111 _ _]
          tunnel: w1097 -> [w1110 _ _]
          tunnel: w1096 -> [w1109 _ _]
          tunnel: w1094 -> [w1106 _ _]
          tunnel: w1093 -> [_ w1184 w1294]
          frame #0 {
            n634 = local read "fab1_totalWt"() -> (w1120:sgl)
            n635 = local read "fab2_totalWt"() -> (w1119:sgl)
            n636 = local read "fab3_totalWt"() -> (w1118:sgl)
            n637 = local read "fab4_totalWt"() -> (w1117:sgl)
            n638 = local read "fab5_totalWt"() -> (w1116:sgl)
            n639 = local read "fab6_totalWt"() -> (w1115:sgl)
            n640 = call "Get Number of Layers (SubVI).vi"("Layers Array"=w1108) -> ("numLayers"=w1107:i32)
            n641 = Format Into String(format string=" VALUES (%d ", w1107) -> (resulting string=w1125:string)  [unwired: 2 in, 1 out]
            n642 = Build Array(w1120, w1119, w1118, w1117, w1116, w1115) -> (w1114:sgl[])
            n643 = for {
              shift-right: [w1135] -> w1112
              shift-left: w1125 -> [w1136]
              shift-right: [w1132] -> w1113
              shift-left: "insert into experiment (plytypes " ("SQL statement") -> [w1133]
              tunnel: w1114 -> [w1126] mode=indexing
              tunnel: w1111 -> [w1131] mode=indexing
              tunnel: w1110 -> [w1130] mode=indexing
              tunnel: w1108 -> [w1128] mode=indexing
              tunnel: w1109 -> [w1129] mode=indexing
              i -> [w1134]
              n644 = Less Or Equal To 0?(x=w1126) -> (x <= 0?=w1127:bool)
              n645 = case shown="False" w1127 {
                tunnel: w1136 -> [w1172 w1175]
                tunnel: [w1171 w1175] -> w1135
                tunnel: w1134 -> [w1170 _]
                tunnel: w1133 -> [w1168 w1174]
                tunnel: [w1167 w1174] -> w1132
                tunnel: w1126 -> [w1161 _]
                tunnel: w1128 -> [w1160 _]
                tunnel: w1131 -> [w1156 _]
                tunnel: w1130 -> [w1155 _]
                tunnel: w1129 -> [w1153 _]
                frame False {
                  # "fabric style"
                  n646 = Unbundle By Name(w1160) -> ("plyNum"=w1146:i32, "LotNum"=w1157:string, "RollNum"=w1158:string, "Fabric.stitch"=w1159:u16)
                  n647 = Unbundle By Name(w1156) -> ("Fabric.fiber"=w1151:string, "Fabric.denier"=w1149:string, "pick"=w1145:string, "weave"=w1150:string, "fabricID_DHB"=w1143:string, "finish"=w1142:string, "SAK_fabric"=w1139:string, "ozPerYd2"=w1141:string)
                  n648 = property on="Fabric.stitch" class="Ring (strict)"() -> ("Strings []"=w1144:string[])  [unwired: 2 in, 2 out]
                  n649 = To Long Integer(number=w1159) -> (32bit integer=w1163:i32)
                  n650 = call <vilib>:"Space Constant.vi"() -> ("String"=w1164:string)
                  n651 = Increment(x=w1170) -> (x+1=w1140:i32)
                  n652 = Index Array(array=w1144, index=w1163) -> (element=w1162:string)
                  n653 = Concatenate Strings(w1157, w1164) -> (w1166:string)
                  n654 = Concatenate Strings(w1158, w1164) -> (w1165:string)
                  n655 = call "Dropdown Selection (SubVI).vi"("reference"=w1153) -> ("element"=w1152:string)
                  n656 = call "Dropdown Selection (SubVI).vi"("reference"=w1155) -> ("element"=w1154:string)
                  n657 = Format Into String(format string=", ply%1dnumber, fab%1d_vendor_PB, fab%1d_styleNum_PB, fab%1d_fiberType_PB, fab%1d_denier_PB, fab%1d_pick_PB, fab%1d_weave_PB, fab%1d_lotNum_PB, fab%1d_rollNum_PB, fab%1d_ozPerYd2_PB,fab%1d_stitch_PB, fab%1d_totalWeight_PB, fab%1d_fabricID_DHB, fab%1d_finishType_PB, FK_styleFabric%1d", initial string=w1168, w1140, w1140, w1140, w1140, w1140, w1140, w1140, w1140, w1140, w1140, w1140, w1140, w1140, w1140, w1140) -> (resulting string=w1167:string)  [unwired: 1 in, 1 out]
                  n658 = Scan From String(input string=w1141, default 1=sgl 0.0 ("default value 1")) -> (output 1=w1148:sgl)  [unwired: 3 in, 3 out]
                  n659 = Scan From String(input string=w1139, default 1=0) -> (output 1=w1138:i32)  [unwired: 3 in, 3 out]
                  n660 = Format Into String(format string=", %d,  '%s',  '%s',  '%s',  '%s',  '%s',  '%s',  '%s',  '%s', %.1f,  '%s', %.2f ,  '%s',  '%s', %d", initial string=w1172, w1146, w1152, w1154, w1151, w1149, w1145, w1150, w1166, w1165, w1148, w1162, w1161, w1143, w1142, w1138) -> (resulting string=w1171:string)  [unwired: 1 in, 1 out]
                }
                frame True {
                }
              }
            }
            n661 = call-poly <vilib>:"DB Tools Open Connection.vi"("connection information"=w1106) -> ("error out"=w1121:errorcluster, "connection reference"=w1122:T20)  [unwired: 7 in]
          }
          frame #1 {
            w1276 = " " ("Substring")
            # "DP/PB shared requirements:"
            # "Added PBBA requirements:"
            n662 = Array Size(array=w1184) -> (size(s)=w1258:i32)
            n663 = local read "Panel"() -> (w1263:i32)
            n664 = local read "currentDateTime"() -> (w1285:string)
            n665 = local read "computed_V50"() -> (w1274:sgl)
            n666 = local read "Drag Corrected"() -> (w1269:bool)
            n667 = local read "Impact factor"() -> (w1271:sgl)
            n668 = local read "Shot Angle"() -> (w1286:u16)
            n669 = Increment(x=w1263) -> (x+1=w1262:i32)
            n670 = control-ref of="ballistician"() -> (w1212:refnum<vi>)
            n671 = control-ref of="Submitter"() -> (w1211:refnum<vi>)
            n672 = control-ref of="Test Conditions"() -> (w1210:refnum<vi>)
            n673 = control-ref of="Type"() -> (w1217:refnum<vi>)
            n674 = control-ref of="Panel Stitch"() -> (w1218:refnum<vi>)
            n675 = control-ref of="Panel Type"() -> (w1219:refnum<vi>)
            n676 = control-ref of="projectileType"() -> (w1201:refnum<vi>)
            n677 = control-ref of="projectileWt"() -> (w1202:refnum<vi>)
            n678 = call "Dropdown Selection (SubVI).vi"("reference"=w1212) -> ("element"=w1209:string)
            n679 = call "Dropdown Selection (SubVI).vi"("reference"=w1211) -> ("element"=w1208:string)
            n680 = call "Dropdown Selection (SubVI).vi"("reference"=w1210) -> ("element"=w1207:string)
            n681 = call "Dropdown Selection (SubVI).vi"("reference"=w1217) -> ("element"=w1216:string)
            n682 = call "Dropdown Selection (SubVI).vi"("reference"=w1218) -> ("element"=w1215:string)
            n683 = call "Dropdown Selection (SubVI).vi"("reference"=w1219) -> ("element"=w1214:string)
            n684 = call "Dropdown Selection (SubVI).vi"("reference"=w1201) -> ("element"=w1179:string)
            n685 = call "Dropdown Selection (SubVI).vi"("reference"=w1202) -> ("element"=w1180:string)
            n686 = local read "totalNumPlies"() -> (w1257:i32)
            n687 = local read "Z.M.R."() -> (w1194:sgl)
            n688 = Select(t=w1271, s=w1269, f=sgl 1.0) -> (s? t:f=w1270:sgl)
            n689 = Equal?(x=w1180, y="Select . . .") -> (x = y?=w1182:bool)
            n690 = Less Than 0?(x=w1194) -> (x < 0?=w1193:bool)
            n691 = Divide(x=w1274, y=w1270) -> (x/y=w1273:sgl)
            n692 = control-ref of="Mfr"() -> (w1231:refnum<vi>)
            n693 = control-ref of="Powder Type"() -> (w1229:refnum<vi>)
            n694 = control-ref of="PanelBack"() -> (w1228:refnum<vi>)
            n695 = control-ref of="N.I.J"() -> (w1226:refnum<vi>)
            n696 = control-ref of="Method"() -> (w1224:refnum<vi>)
            n697 = control-ref of="PanelDim"() -> (w1223:refnum<vi>)
            n698 = Concatenate Strings(w1216, w1276, w1215, w1276, w1214, w1276, "Fabric Description") -> (w1250:string)
            n699 = case shown="False" w1182 {
              tunnel: [w1287 "0" ("element")] -> w1181
              tunnel: w1180 -> [w1287 _]
              frame False {
              }
              frame True {
              }
            }
            n700 = case shown="True" w1193 {
              tunnel: w1194 -> [w1292 _]
              tunnel: [w1292 sgl 0.0 ("Z.M.R.")] -> w1192
              frame False {
              }
              frame True {
              }
            }
            n701 = call "Dropdown Selection (SubVI).vi"("reference"=w1231) -> ("element"=w1230:string)
            n702 = call "Dropdown Selection (SubVI).vi"("reference"=w1229) -> ("element"=w1178:string)
            n703 = call "Dropdown Selection (SubVI).vi"("reference"=w1228) -> ("element"=w1227:string)
            n704 = call "Dropdown Selection (SubVI).vi"("reference"=w1226) -> ("element"=w1225:string)
            n705 = call "Dropdown Selection (SubVI).vi"("reference"=w1224) -> ("element"=w1185:string)
            n706 = call "Dropdown Selection (SubVI).vi"("reference"=w1223) -> ("element"=w1222:string)
            n707 = control-ref of="Panel Technician"() -> (w1221:refnum<vi>)
            n708 = call "Dropdown Selection (SubVI).vi"("reference"=w1221) -> ("element"=w1220:string)
            n709 = Equal?(x=w1185, y="V50") -> (x = y?=w1187:bool)
            n710 = local read "rangeOfResults"() -> (w1176:i32)
            n711 = case shown="True" w1187 {
              tunnel: ["n/a" w1291] -> w1186
              frame False {
              }
              frame True {
                n712 = Format Into String("minV50") -> (resulting string=w1291:string)  [unwired: 3 in, 1 out]
              }
            }
            n713 = local read "totalBAW"() -> (w1213:sgl)
            n714 = local read "threatDetails"() -> (w1199:T2)
            n715 = control-ref of="standard"() -> (w1249:refnum<vi>)
            n716 = control-ref of="workType"() -> (w1191:refnum<vi>)
            n717 = control-ref of="Model"() -> (w1189:refnum<vi>)
            n718 = local read "lowComplete"() -> (w1177:i32)
            n719 = control-ref of="projectileType"() -> (w1232:refnum<vi>)
            n720 = call "Dropdown Selection (SubVI).vi"("reference"=w1249) -> ("element"=w1248:string)
            n721 = call "Dropdown Selection (SubVI).vi"("reference"=w1191) -> ("element"=w1245:string)
            n722 = call "Dropdown Selection (SubVI).vi"("reference"=w1189) -> ("element"=w1190:string)
            n723 = control-ref of="covering"() -> (w1242:refnum<vi>)
            n724 = call "Dropdown Selection (SubVI).vi"("reference"=w1232) -> ("element"=w1233:string)
            n725 = control-ref of="shooter"() -> (w1240:refnum<vi>)
            n726 = control-ref of="recorder"() -> (w1238:refnum<vi>)
            n727 = control-ref of="rangeNum"() -> (w1205:refnum<vi>)
            n728 = control-ref of="weapon"() -> (w1235:refnum<vi>)
            n729 = local read "clayAverage"() -> (w1196:sgl)
            n730 = Unbundle By Name(w1199) -> ("barrelLength"=w1200:string, "FK_threat"=w1195:string)
            n731 = local read "highPartial"() -> (w1206:i32)
            n732 = call "Dropdown Selection (SubVI).vi"("reference"=w1242) -> ("element"=w1241:string)
            n733 = call "Dropdown Selection (SubVI).vi"("reference"=w1240) -> ("element"=w1239:string)
            n734 = call "Dropdown Selection (SubVI).vi"("reference"=w1238) -> ("element"=w1237:string)
            n735 = call "Dropdown Selection (SubVI).vi"("reference"=w1205) -> ("element"=w1204:string)
            n736 = call "Dropdown Selection (SubVI).vi"("reference"=w1235) -> ("element"=w1234:string)
            n737 = Scan From String(input string=w1195, default 1=0) -> (output 1=w1197:i32)  [unwired: 3 in, 3 out]
            n738 = Format Into String(format string=", %d, #%s#, '%s', '%s', %d, '%s', '%s', %.4f, '%s', '%s', '%s', %.4f, %.1f, %.6f, '%s', %.4f, '%s', %d, '%s', %d, '%s', '%s', %d, '%s', %d, %d, %.2f, '%s', %.1f, '%s', '%s', '%s', '%s', '%s', '%s', '%s', '%s', %.1f, %.1f, '%s', '%s', '%s', '%s', '%s', '%s', '%s', '%s', %d, '%s', %.1f, %d, %d, %d, %d)" ("Format String"), initial string=w1278, w1262, w1285, w1209, w1208, w1286, w1207, w1250, "Areal Density", "Areal density text", w1179, w1181, "Weight of Panel", w1274, w1273, w1230, "Thickness", w1178, w1258, w1227, w1257, "Comments", w1225, "B.F.S (mm)", w1185, "RoomT", "RoomHum", "Version", w1222, w1192, "Sample #", w1220, w1248, "projName", "projNum", w1245, "serialNum", w1190, "totalSampleWt", w1213, w1241, w1186, w1239, w1237, w1204, w1234, w1233, w1200, "clayTemp", "clayCalib", w1196, w1206, w1177, w1176, w1197) -> (resulting string=w1277:string)  [unwired: 1 in, 1 out]
            n739 = Concatenate Strings(w1284, ", expt, [date], operator, submitter, angle, conditions, fabric, density, densitytext, threat,weight, panelweight, v50dc, v50 , maker, thickness, powder, numshots, backing, totalnumberplys, testcomments, nij, bfs, method, temperature, humidity, version, dimensions, zmr, sampleid, panelmaker,\nstandard_PB, projName_PB, projNum_PB, workType_PB, serialNum_PB, model_PB, totalSampleWt_PB,totalBAW_PB,covering_PB, minV50_PB,  shooter_PB, recorder_PB, rangeNum_PB, weapon_PB, projectile_PB, barrelLen_PB, clayTemp_PB, clayCal_PB, clayAvg_PB, highPartial_PB, lowComplete_PB, rangeOfResults_PB,FK_Projectile)" ("Substring"), w1277) -> (w1268:string)
            n740 = call-poly <vilib>:"DB Tools Execute Query.vi"("error in (no error)"=w1260, "SQL query"=w1268, "connection reference"=w1261) -> ("error out"=w1267:errorcluster, "recordset reference"=w1265:T21)  [unwired: 5 in]
            n741 = call-poly <vilib>:"DB Tools Free Object.vi"("error in (no error)"=w1267, "recordset reference"=w1265) -> ("error out"=w1266:errorcluster, "connection reference"=w1264:T20)  [unwired: 8 in]
          }
          frame #2 {
            # "Experiment.expt"
            n742 = local read "Shot"() -> (w1301:i32)
            n743 = Increment(x=w1301) -> (x+1=w1299:i32)
            n744 = for {
              tunnel: w1294 -> [w1347] mode=indexing
              tunnel: w1303 -> [w1319]
              tunnel: w1302 -> [w1321]
              tunnel: [w1317] -> w1296
              tunnel: [w1318] -> w1298
              tunnel: w1299 -> [w1325]
              tunnel: [w1316] -> w1300
              tunnel: w1295 -> [w1312]
              i -> [w1316]
              # "Shot.id"
              n745 = Add(x=w1325, y=w1316) -> (x+y=w1324:i32)
              n746 = local read "Drag Corrected"() -> (w1305:bool)
              n747 = local read "Residual factor"() -> (w1330:sgl)
              n748 = local read "Impact factor"() -> (w1304:sgl)
              n749 = Unbundle By Name(w1347) -> ("IMPACT VELOCITY"=w1333:sgl, "Redundant_Velocity"=w1308:sgl, "RESIDUAL  VELOCITY"=w1307:sgl, "Shot Description"=w1309:string, "Powder Loading"=w1337:sgl, "Barrel Temperature"=w1338:sgl, "TIME / DATE"=w1339:string, "shot order"=w1340:i32, "Shot Angle"=w1341:u16, "BackFace\nDepth"=w1342:sgl, "BackFace\nDiameter"=w1343:sgl, "SHOT STATUS"=w1345:u16, "Projectile Mass"=w1336:sgl, "usedv50"=w1335:bool, "Energy Loss (J)"=w1334:sgl, "avgVel_PB"=w1315:sgl, "velLoss_PB"=w1314:sgl, "strikeVel_PB"=w1313:sgl)
              n750 = Select(t=w1304, s=w1305, f=sgl 1.0) -> (s? t:f=w1328:sgl)
              n751 = Select(t=w1304, s=w1305, f=sgl 1.0) -> (s? t:f=w1310:sgl)
              n752 = Select(t=w1330, s=w1305, f=sgl 1.0) -> (s? t:f=w1329:sgl)
              n753 = Greater Than 0?(x=w1345) -> (x > 0?=w1344:bool)
              n754 = Divide(x=w1333, y=w1328) -> (x/y=w1326:sgl)
              n755 = Divide(x=w1308, y=w1310) -> (x/y=w1306:sgl)
              n756 = Divide(x=w1307, y=w1329) -> (x/y=w1332:sgl)
              n757 = Format Into String(format string="INSERT INTO shots (impactdc, redundantdc, residualdc,  comment, loading, barreltemp, [date], [order], shotangle, bfdepth, bfdiameter, [complete], expt, id, weight,usedv50, loss, residual, impact, redundant, avgVel_PB, velLoss_PB, strikeVel_PB)  VALUES (%.1f, %.1f, %.1f, '%s', %.4f, %.1f, #%s#, %d, %d, %.3f, %.3f, %d, %d, %d, %.4f, %d, %.4f, %.1f, %.1f, %.1f, %.1f, %.1f, %.1f)" ("Substring"), w1333, w1308, w1307, w1309, w1337, w1338, w1339, w1340, w1341, w1342, w1343, w1344, w1312, w1324, w1336, w1335, w1334, w1332, w1326, w1306, w1315, w1314, w1313) -> (resulting string=w1320:string)  [unwired: 2 in, 1 out]
              n758 = call-poly <vilib>:"DB Tools Execute Query.vi"("error in (no error)"=w1321, "SQL query"=w1320, "connection reference"=w1319) -> ("error out"=w1323:errorcluster, "recordset reference"=w1322:T21)  [unwired: 5 in]
              n759 = call-poly <vilib>:"DB Tools Free Object.vi"("error in (no error)"=w1323, "recordset reference"=w1322) -> ("error out"=w1317:errorcluster, "connection reference"=w1318:T20)  [unwired: 8 in]
            }
            n760 = call <vilib>:"DB Tools Close Connection.vi"("error in (no error)"=w1296, "connection reference"=w1298) -> ("error out"=w1297:errorcluster)  [unwired: 5 in]
          }
        }
        n761 = case shown="No Error" w1101 {
          selector: w1101 -> [w1352 w1369]
          tunnel: [w1351 w1371] -> w1104
          tunnel: [w1351 w1371] -> w1105
          tunnel: w1103 -> [w1364 _]
          tunnel: w1095 -> [w1353 _]
          frame No Error {
            w1354 = "Data Base Parameters" ("section")
            w1351 = 6
            n762 = local read "Shot"() -> (w1365:i32)
            n763 = Increment(x=w1365) -> (x+1=w1359:i32)
            n764 = call <vilib>:"Open Config Data (compatibility).vi"("error in (no error)"=w1352, "configuration file path"=w1353) -> ("error out"=w1358:errorcluster, "refnum"=w1357:T22)  [unwired: 7 in, 1 out]
            n765 = Add(x=w1359, y=w1364) -> (x+y=w1360:i32)
            n766 = flat-sequence {
              tunnel: w1350 -> [_]
              frame #0 {
                w1366 = u8 2 ("Disabled")
                n767 = One Button Dialog(message="Data Saved") -> ()  [unwired: 1 in, 1 out]
                n768 = property on="Clear" class="Bool"("Disabled"=u8 0) -> ()  [unwired: 2 in, 2 out]
                n769 = property on="Accept Data" class="Bool (strict)"("Disabled"=w1366) -> ()  [unwired: 2 in, 2 out]
                n770 = property on="Reject shot" class="Bool"("Disabled"=w1366) -> ()  [unwired: 2 in, 2 out]
                n771 = property on="Save" class="Bool"("Disabled"=w1366) -> ()  [unwired: 2 in, 2 out]
              }
            }
            n772 = local write "Shot"(w1360) -> ()
            n773 = local read "Panel"() -> (w1361:i32)
            n774 = call-poly <vilib>:"Write Key.vi"("section"=w1354, "error in (no error)"=w1358, "value"=w1360, "key"="Last Shot Saved ", "refnum"=w1357) -> ("error out"=w1356:errorcluster, "refnum out"=w1355:T22)  [unwired: 4 in, 1 out]
            n775 = Increment(x=w1361) -> (x+1=w1348:i32)
            n776 = local write "Panel"(w1348) -> ()
            n777 = call-poly <vilib>:"Write Key.vi"("section"=w1354, "error in (no error)"=w1356, "value"=w1348, "key"="Last Panel Saved ", "refnum"=w1355) -> ()  [unwired: 4 in, 3 out]
            n778 = To Double Precision Float(number=w1348) -> (double precision float=w1349:dbl)
            n779 = call <vilib>:"Close Config Data.vi"("error in (no error)"=w1356, "refnum"=w1355) -> ("error out"=w1350:errorcluster)  [unwired: 8 in, 1 out]
            n780 = property on="Record #" class="DigNum (strict)"("Maximum"=w1349) -> ()  [unwired: 2 in, 2 out]
          }
          frame Error {
            w1371 = -1
            n781 = call <vilib>:"Simple Error Handler.vi"("error in (no error)"=w1369) -> ()  [unwired: 4 in, 5 out]
            n782 = One Button Dialog(message="Error saving Data. ") -> ()  [unwired: 1 in, 1 out]
          }
        }
      }
      frame 5 {
        w1414 = -1 ("index of element")
        # "ACCEPT DATA"
        # "Shot Order"
        # "This section accepts new data to the shot table."
        n783 = local read "residual/speed"() -> (w1390:sgl)
        n784 = local read "Impact/speed"() -> (w1385:sgl)
        n785 = Not(x=w1377) -> (.not. x?=w1376:bool)
        n786 = property on="Reject shot" class="Bool"("Disabled"=u8 0) -> ()  [unwired: 2 in, 2 out]
        n787 = local read "Current/redundant/speed"() -> (w1383:sgl)
        n788 = local read "Current/residual/speed"() -> (w1404:sgl)
        n789 = local read "Current/impact/speed"() -> (w1382:sgl)
        n790 = local read "BACKFACE DIAMETER"() -> (w1409:sgl)
        n791 = local read "Corrected Redundant"() -> (w1380:sgl)
        n792 = local read "Current/avg/speed"() -> (w1378:sgl)
        n793 = local read "Corrected Residual"() -> (w1405:sgl)
        n794 = Array Size(array=w1375) -> (size(s)=w1407:i32)
        n795 = local read "BACKFACE DEPTH"() -> (w1401:sgl)
        n796 = local read "Redundant/speed"() -> (w1381:sgl)
        n797 = local read "Corrected Impact"() -> (w1403:sgl)
        n798 = local read "conversion factor"() -> (w1393:sgl)
        n799 = local read "SHOT STATUS"() -> (w1408:u16)
        n800 = local read "Avg/speed"() -> (w1379:sgl)
        n801 = Increment(x=w1407) -> (x+1=w1384:i32)
        n802 = local write "Accept Data"(FALSE) -> ()
        n803 = Multiply(x=w1385, y=w1393) -> (x*y=w1395:sgl)
        n804 = Multiply(x=w1393, y=w1390) -> (x*y=w1394:sgl)
        n805 = Multiply(x=w1395, y=w1395) -> (x*y=w1400:sgl)
        n806 = Multiply(x=w1394, y=w1394) -> (x*y=w1399:sgl)
        n807 = Subtract(x=w1400, y=w1399) -> (x-y=w1397:sgl)
        n808 = Format Date/Time String(time format string (%c)="%x   %H:%M:%S") -> (date/time string=w1389:string)  [unwired: 2 in]
        "SUBMIT DATE/TIME" <- w1389
        n809 = Compound Arithmetic op=MULTIPLY("Projectile Mass", w1397, sgl 0.0005 ("Input")) -> (w1392:sgl)
        n810 = Index Array(array=w1375) -> (element=w1410:T5)  [unwired: 1 in]
        n811 = Bundle By Name(cluster=w1410, "TIME / DATE"=w1389, "shot order"=w1384, "IMPACT VELOCITY"=w1385, "RESIDUAL  VELOCITY"=w1390, "Shot Description"="Shot Decription", "Powder Loading"="Powder Loading", "Barrel Temperature"="Barrel Temp", "SHOT STATUS"=w1408, "BackFace\nDepth"=w1401, "BackFace\nDiameter"=w1409, "Shot Angle"="Shot Angle", "Uncorrected Impact"=w1382, "Corrected Impact"=w1403, "Uncorrected Residual"=w1404, "Corrected residual"=w1405, "Projectile Mass"="Projectile Mass", "Energy Loss (J)"=w1392, "UncorrectedRed_PB"=w1383, "Redundant_Velocity"=w1381, "CorrectedRed_PB"=w1380, "UncorrectedAvgVel_PB"=w1378, "avgVel_PB"=w1379) -> (w1406:T5)
        n812 = Build Array (concatenate)(w1375, w1406) -> (w1374:T5[])
      }
      frame 6 {
        w1418 = u8 2 ("Disabled")
        w1420 = -1
        # "This section will clear the shot table and re-enable the \"ADD SHOT\" button to get ready for a new test panel."
        # "CLEAR SHOTS"
        n813 = invoke on="Table of Shots" class="Tbl (strict)" method="Reinit To Default"() -> ()  [unwired: 3 in, 3 out]
        n814 = invoke on="SHOTS" class="Arr (strict)" method="Reinit To Default"() -> ()  [unwired: 3 in, 3 out]
        n815 = property on="Accept Data" class="Bool (strict)"("Disabled"=u8 0) -> ()  [unwired: 2 in, 2 out]
        n816 = property on="Clear" class="Bool"("Disabled"=w1418) -> ()  [unwired: 2 in, 2 out]
        n817 = property on="Reject shot" class="Bool"("Disabled"=w1418) -> ()  [unwired: 2 in, 2 out]
        n818 = property on="Save" class="Bool"("Disabled"=w1418) -> ()  [unwired: 2 in, 2 out]
      }
      frame 7 {
        w1430 = -1
        # "REJECT LAST SHOT OR DELETE SHOT RECORD"
        # "This section unaccepts new data  OR deletes the currently accessed previous shot"
        n819 = local read "Delete Button"() -> (w1429:bool)
        n820 = case shown="True" w1429 {
          tunnel: w1428 -> [w1433 w1445]
          tunnel: [w1434 w1446] -> w1425
          frame False {
            n821 = Array Size(array=w1433) -> (size(s)=w1431:i32)
            n822 = local write "SUBMIT DATE/TIME"("" ("Empty String Constant")) -> ()
            n823 = while {
              tunnel: [w1437] -> w1432
              tunnel: w1431 -> [w1439]
              tunnel: w1433 -> [w1441] mode=indexing
              i -> [w1437]
              stop <- w1440 stop-if-true
              n824 = Unbundle By Name(w1441) -> ("shot order"=w1438:i32)
              n825 = Equal?(x=w1438, y=w1439) -> (x = y?=w1440:bool)
            }
            n826 = Delete From Array "Delete From Array"(array=w1433, index=w1432) -> (array with subset deleted=w1434:T5[])  [unwired: 1 in, 1 out]
            n827 = property on="Reject shot" class="Bool"("Disabled"=u8 2) -> ()  [unwired: 2 in, 2 out]
          }
          frame True {
            n828 = property on="SHOTS" class="Arr (strict)"() -> ("Index Values"=w1454:u32[])  [unwired: 2 in, 2 out]
            n829 = local write "Delete Button"(FALSE) -> ()
            n830 = Index Array(array=w1454, index=0 ("Index")) -> (element=w1444:u32)
            n831 = Index Array(array=w1445, index=w1444) -> (element=w1443:T5)
            n832 = Unbundle By Name(w1443) -> ("shot order"=w1442:i32)
            n833 = Format Into String(format string="The currently displayed Shot, #%d", w1442) -> (resulting string=w1451:string)  [unwired: 2 in, 1 out]
            n834 = Concatenate Strings(w1451, ", will be deleted.  IT CANNOT RECOVERED!  Do you want to DELETE the shot?" ("message")) -> (w1450:string)
            n835 = Two Button Dialog(message=w1450, 1:"NO I do NOT want to delete.  Cancel Request" ("F button name (\"Cancel\")"), 2:"YES I want to delete the shot" ("T button name (\"OK\")")) -> (T button?=w1457:bool)
            n836 = case shown="True" w1457 {
              tunnel: w1445 -> [w1470 w1473]
              tunnel: [w1470 w1475] -> w1448
              tunnel: w1444 -> [_ w1472]
              tunnel: [10000 ("shot order") w1474] -> w1447
              frame False {
              }
              frame True {
                n837 = Index Array(array=w1473, index=w1472) -> (element=w1471:T5)
                n838 = Unbundle By Name(w1471) -> ("shot order"=w1474:i32)
                n839 = Delete From Array(array=w1473, index=w1472) -> (array with subset deleted=w1475:T5[])  [unwired: 1 in, 1 out]
              }
            }
            n840 = for {
              tunnel: [w1464] -> w1446 mode=indexing
              tunnel: w1448 -> [w1459] mode=indexing
              tunnel: w1447 -> [w1463]
              n841 = Unbundle By Name(w1459) -> ("shot order"=w1461:i32)
              n842 = Decrement(x=w1461) -> (x-1=w1460:i32)
              n843 = Greater?(x=w1461, y=w1463) -> (0:w1462:bool)
              n844 = case shown="True" w1462 {
                tunnel: w1460 -> [_ w1467]
                tunnel: w1459 -> [w1465 w1468]
                tunnel: [w1465 w1466] -> w1464
                frame False {
                }
                frame True {
                  n845 = Bundle By Name(cluster=w1468, "shot order"=w1467) -> (w1466:T5)
                }
              }
            }
          }
        }
        n846 = property on="SHOTS" class="Arr (strict)"("Val(Sgnl)"=w1425) -> ()  [unwired: 2 in, 2 out]
      }
      frame 8 {
        w1487 = -1
        # "RESET RANGE"
        # "This section will reset range"
        n847 = Concatenate Strings("L|", "6|") -> (w1481:string)
        n848 = case shown="2" "Data Source" {
          tunnel: [w1488 w1491 w1494] -> w1483
          tunnel: w1482 -> [w1488 w1491 w1493]
          tunnel: w1481 -> [_ _ w1492]
          frame 0, Default {
            n849 = flat-sequence {
              frame #0 {
                n850 = local write "RANGE RESET"(FALSE ("RANGE RESET")) -> ()
              }
              frame #1 {
                n851 = Wait (ms)(milliseconds to wait=u32 100) -> ()  [unwired: 1 out]
              }
            }
          }
          frame 1 {
          }
          frame 2 {
            w1502 = u32 22 items=["NI-DAQ version", "device name", "base address", "data transfer mode for analog input", "data transfer mode for analog output group 1", "data transfer mode for analog output group 2", "data transfer mode for GPCTR 0", "data transfer mode for GPCTR 1", "data transfer mode for digital I/O group 1", "data transfer mode for digital I/O group 2", "device type code", "DMA A level", "DMA B level", "DMA C level", "interrupt A level", "interrupt B level", "reserved", "lpt device mode", "DAQCard-700 counter 1 source", "interrupt generation mode", "device state during suspend mode", "computer name", "serial number", "counter type", "Scarab A Memory Size", "Scarab B Memory Size"] ("information type")
            w1501 = u32 1  # device
            # "Screens"
            n852 = Concatenate Strings(w1492, "2|") -> (w1497:string)
            n853 = call "Get DAQ Device Information.vi"("information type"=w1502, "task ID or device"=w1501) -> ("error out"=w1496:errorcluster, "information string"=w1500:string)  [unwired: 7 in, 1 out]
            n854 = disable-structure "Diagram Disable Structure" shown="Disabled" {
              disable-tunnel: w1497 -> [w1508 _]
              disable-tunnel: w1496 -> [w1505 w1510]
              disable-tunnel: [w1504 w1510] -> w1495
              frame Disabled {
                n855 = Current VI's Path() -> (path=w1509:path)
                n856 = call "Where Am I (SubVI).vi"("TL Calling Location"=w1508, "Call VI path"=w1509) -> ("I'm here"=w1507:string)
                n857 = call "Error Check (SubVI).vi"("calling VI"=w1507, "tag #"=0, "error IN"=w1505) -> ("error OUT"=w1504:errorcluster)  [unwired: 2 in]
              }
              frame Enabled {
                # "Debug code is disabled"
              }
            }
            n858 = Unbundle By Name(w1496) -> ("status"=w1503:bool)
            n859 = case shown="True" w1503 {
              tunnel: w1500 -> [w1520 _]
              tunnel: [w1520 "DEVICE NOT READY!" ("information string")] -> w1499
              tunnel: w1495 -> [w1519 _]
              tunnel: [w1512 w1525] -> w1494
              tunnel: w1493 -> [_ w1525]
              frame False {
                # "assign task IDs to counters"
                n860 = local write "RANGE RESET"(FALSE ("RANGE RESET")) -> ()
                n861 = call "Config Counter to Measure Two Edge Separation.vi"("error IN"=w1519, "Counter"="Impact Timer", "device"="DAQ Card") -> ("error out"=w1522:errorcluster, "task ID out"=w1515:u32)  [unwired: 1 in]
                "impact/ID" <- w1515
                n862 = call "Config Counter to Measure Two Edge Separation.vi"("error IN"=w1522, "Counter"="Residual  Timer", "device"="DAQ Card") -> ("error out"=w1524:errorcluster, "task ID out"=w1513:u32)  [unwired: 1 in]
                "residual/ID" <- w1513
                n863 = call "Config Counter to Measure Two Edge Separation.vi"("error IN"=w1524, "Counter"="Redundant Timer", "device"="DAQ Card") -> ("error out"=w1523:errorcluster, "task ID out"=w1514:u32)  [unwired: 1 in]
                "Red/ID" <- w1514
                n864 = Bundle("task ID out"=w1515, "task ID out"=w1514, "task ID out"=w1513) -> (w1512:T23)  [unwired: 1 in]
                n865 = call <vilib>:"Simple Error Handler.vi"("error in (no error)"=w1523) -> ()  [unwired: 4 in, 5 out]
              }
              frame True {
                w1528 = u16 0 items=["Simulated", "Radar", "Screens"] ("Data Source")
                n866 = local write "Data Source"(w1528) -> ()
                n867 = One Button Dialog(message="Error initializing Timer board.  Switching to simulation") -> ()  [unwired: 1 in, 1 out]
              }
            }
            "Device S/N" <- w1499
          }
        }
        n868 = local write "SUBMIT DATE/TIME"("" ("Empty String Constant")) -> ()
      }
    }
  }
  n869 = while {
    shift-right: [w1529] -> _
    shift-left: "" ("NewVal") -> [w1530]
    stop <- FALSE stop-if-true
    n870 = event shown="[12] \"Method\": Value Change" {
      selector: _ -> [_ _ _ _ _ _ _ _ _ _ _ _ _]
      dyn-events: _ -> [_ _ _ _ _ _ _ _ _ _ _ _ _]
      timeout: _ -> [_ _ _ _ _ _ _ _ _ _ _ _ _]
      tunnel: w1530 -> [w1532 _ w1534 w1537 w1554 w1571 w1584 w1617 w1656 w1660 w1697 w1729 w1731]
      tunnel: [w1532 w1533 w1534 w1537 w1554 w1571 w1584 w1617 w1656 w1660 w1697 w1729 w1731] -> w1529
      event Timeout {
        n871 = event-data() -> ()  [unwired: 1 in, 2 out]
      }
      event "connStr": Value Change {
        n872 = event-data() -> ("NewVal"=w1533:string)  [unwired: 1 in, 5 out]
      }
      event "projectileType": Value Change {
        n873 = event-data() -> ()  [unwired: 1 in, 6 out]
        n874 = control-ref of="projectileType"() -> (w1536:refnum<vi>)
        n875 = call "Get Projectile Atributes.vi"("connectString"=w1534, "projectile"=w1536) -> ("projectileAttribs"=→"threatDetails":T2)
      }
      event "projectileWt": Value Change {
        n876 = event-data() -> ("CtlRef"=w1546:refnum<vi>)  [unwired: 1 in, 5 out]
        n877 = property on="Property Node" class="Ring (strict)"(reference=w1546) -> (reference out=w1541:refnum<vi>, "RingText.Text"=w1545:string)  [unwired: 1 in, 1 out]
        n878 = call "Select Projectile Type.vi"("connectString"=w1537, "projectileWeight"=w1545) -> ("projectileTypes"=w1544:string[])
        n879 = property on="projectileType" class="Ring (strict)"("Strings []"=w1544, "Val(Sgnl)"=u16 0 ("Value (Signaling)")) -> ()  [unwired: 2 in, 2 out]
        n880 = call "Dropdown Selection (SubVI).vi"("reference"=w1541) -> ("element"=w1540:string)
        n881 = Equal?(x=w1540, y="Select . . .") -> (x = y?=w1538:bool)
        n882 = case shown="False" w1538 {
          tunnel: [w1550 sgl 0.0] -> w1542
          tunnel: w1540 -> [w1547 _]
          frame False {
            w1552 = sgl 0.0  # sgl
            n883 = Scan From String(format string="%f " ("Format String"), input string=w1547, default 1=w1552) -> (output 1=w1551:sgl)  [unwired: 2 in, 3 out]
            n884 = Multiply(x=sgl 0.06479891, y=w1551) -> (x*y=w1550:sgl)
          }
          frame True {
          }
        }
        n885 = local write "Projectile Mass"(w1542) -> ()
      }
      event "fabVendor_1", "fabVendor_2", "fabVendor_3", "fabVendor_4", "fabVendor_5", "fabVendor_6": Value Change {
        n886 = event-data() -> ("CtlRef"=w1562:refnum<vi>)  [unwired: 1 in, 5 out]
        n887 = property on="Property Node" class="Ring (strict)"(reference=w1562) -> ("Label.Text"=w1558:string, "RingText.Text"=w1559:string)  [unwired: 1 in, 2 out]
        n888 = call "Select Fabric Style.vi"("connectString"=w1554, "Vendor"=w1559) -> ("fabStyles"=w1563:string[])
        n889 = Scan From String(format string="fabVendor_%d", input string=w1558, default 1=0 ("default value 1")) -> (output 1=w1557:i32)  [unwired: 2 in, 3 out]
        n890 = case shown="1" w1557 {
          tunnel: [refnum<vi> refnum ("fabStyle_6") w1565 w1566 w1567 w1568 w1569 w1570] -> w1556
          frame 0, Default {
          }
          frame 1 {
            n891 = control-ref of="fabStyle_1"() -> (w1565:refnum<vi>)
          }
          frame 2 {
            n892 = control-ref of="fabStyle_2"() -> (w1566:refnum<vi>)
          }
          frame 3 {
            n893 = control-ref of="fabStyle_3"() -> (w1567:refnum<vi>)
          }
          frame 4 {
            n894 = control-ref of="fabStyle_4"() -> (w1568:refnum<vi>)
          }
          frame 5 {
            n895 = control-ref of="fabStyle_5"() -> (w1569:refnum<vi>)
          }
          frame 6 {
            n896 = control-ref of="fabStyle_6"() -> (w1570:refnum<vi>)
          }
        }
        n897 = property class="Ring (strict)"(reference=w1556, "Strings []"=w1563, "Val(Sgnl)"=u16 0 ("Value (Signaling)")) -> ()  [unwired: 1 in, 2 out]
      }
      event "fabStyle_1", "fabStyle_2", "fabStyle_3", "fabStyle_4", "fabStyle_5", "fabStyle_6": Value Change {
        n898 = event-data() -> ("CtlRef"=w1577:refnum<vi>)  [unwired: 1 in, 5 out]
        n899 = call "Get Fabic Style Atributes.vi"("connectString"=w1571, "Ring Refnum"=w1577) -> ("projectileAttribs"=w1572:T24)
        n900 = property class="Ring (strict)"(reference=w1577) -> ("Label.Text"=w1576:string)  [unwired: 1 in, 2 out]
        n901 = Scan From String(format string="fabStyle_%d", input string=w1576, default 1=0 ("default value 1")) -> (output 1=w1574:i32)  [unwired: 2 in, 3 out]
        n902 = case shown="1" w1574 {
          tunnel: w1572 -> [_ w1578 w1579 w1580 w1581 w1582 w1583]
          frame 0, Default {
          }
          frame 1 {
            n903 = property on="fabAttribs_1" class="Clust (strict)"("Val(Sgnl)"=w1578) -> ()  [unwired: 2 in, 2 out]
            "fabAttribs_1" <- w1578
          }
          frame 2 {
            n904 = property on="fabAttribs_2" class="Clust (strict)"("Val(Sgnl)"=w1579) -> ()  [unwired: 2 in, 2 out]
            "fabAttribs_2" <- w1579
          }
          frame 3 {
            n905 = property on="fabAttribs_3" class="Clust (strict)"("Val(Sgnl)"=w1580) -> ()  [unwired: 2 in, 2 out]
            "fabAttribs_3" <- w1580
          }
          frame 4 {
            n906 = property on="fabAttribs_4" class="Clust (strict)"("Val(Sgnl)"=w1581) -> ()  [unwired: 2 in, 2 out]
            "fabAttribs_4" <- w1581
          }
          frame 5 {
            n907 = property on="fabAttribs_5" class="Clust (strict)"("Val(Sgnl)"=w1582) -> ()  [unwired: 2 in, 2 out]
            "fabAttribs_5" <- w1582
          }
          frame 6 {
            n908 = property on="fabAttribs_6" class="Clust (strict)"("Val(Sgnl)"=w1583) -> ()  [unwired: 2 in, 2 out]
            "fabAttribs_6" <- w1583
          }
        }
      }
      event "velocity-loading": Value Change {
        w1592 = FALSE ("Visible")
        w1593 = TRUE ("Visible")
        w1602 = "" ("replace string (\"\")")
        # "This section plots  Impact velocity vs. loadingdata"
        n909 = event-data() -> ()  [unwired: 1 in, 6 out]
        n910 = invoke on="v50 data 2" class="Tbl" method="Reinit To Default"() -> (error out=w1589:errorcluster)  [unwired: 3 in, 2 out]
        n911 = call "Trim String.vi"("inStr"="Powder") -> ("outStr"=w1600:string)
        n912 = call "Trim String.vi"("inStr"="Threat") -> ("outStr"=w1601:string)
        n913 = invoke on="Velocity versus Loading" class="XYGraph (strict)" method="Reinit To Default"(error in=w1589) -> (error out=w1588:errorcluster)  [unwired: 2 in, 2 out]
        n914 = property on="Data retrieval" class="Str"(error in=w1588, "Visible"=w1593, "Blinking"=w1593) -> (error out=w1590:errorcluster)  [unwired: 1 in, 1 out]
        n915 = Format Into String(format string="  select top %d experiment.threat,  shots.loading, shots.impact,  experiment.powder, shots.date from shots, experiment where shots.expt = experiment.expt and shots.loading > .02 and shots.date between  #%s# and #%s# and shots.impact between 5000 and 10 and experiment.powder like '%%%s%%' and experiment.threat like '%%%s%%' and experiment.threat<>'' order by experiment.threat, shots.loading,shots.impact" ("Format String"), error in=w1590, "maxRecs", "Earliest Date", "latest Date", w1600, w1601) -> (resulting string=w1606:string, error out=w1586:errorcluster)  [unwired: 1 in]
        n916 = Search and Replace String(input string=w1606, search string=" and experiment.powder like '%%'", replace string=w1602, error in=w1586) -> (result string=w1604:string, error out=w1587:errorcluster)  [unwired: 4 in, 2 out]
        n917 = Search and Replace String(input string=w1604, search string="and experiment.threat like '%%'", replace string=w1602, error in=w1587) -> (result string=w1595:string, error out=w1585:errorcluster)  [unwired: 4 in, 2 out]
        n918 = call "Fetch Data (SubVI).vi"("error IN"=w1585, "connectString"=w1584, "query string"=w1595) -> ("error OUT"=w1591:errorcluster, "recordset data"=w1596:string[][])
        "v50 data 2" <- w1596
        n919 = property on="Data retrieval" class="Str"(error in=w1591, "Visible"=w1592, "Blinking"=w1592) -> ()  [unwired: 1 in, 2 out]
        n920 = Fract/Exp String To Number(string=w1596) -> (number=w1610:dbl[][])  [unwired: 3 in, 1 out]
        n921 = Array Size(array=w1596) -> (size(s)=w1598:i32[])
        n922 = Index Array(array=w1598) -> (element=→"ActualNumRecs":i32)  [unwired: 1 in]
        n923 = Index Array(array=w1610, index (col)=2 ("Disabled Index (col)")) -> (element=w1609:dbl[])  [unwired: 1 in]
        n924 = Index Array(array=w1610, index (col)=1 ("Disabled Index (col)")) -> (element=w1608:dbl[])  [unwired: 1 in]
        n925 = Bundle(w1608, w1609) -> (→"Velocity versus Loading":cluster{dbl[], dbl[]})  [unwired: 1 in]
      }
      event "Panel Search": Value Change {
        # "This section plots panel V50 data"
        n926 = event-data() -> ()  [unwired: 1 in, 6 out]
        n927 = invoke on="v50 data" class="Tbl" method="Reinit To Default"() -> (error out=w1631:errorcluster)  [unwired: 3 in, 2 out]
        n928 = invoke on="Previous V50 Data" class="WFGraph (strict)" method="Reinit To Default"(error in=w1631) -> (error out=w1630:errorcluster)  [unwired: 2 in, 2 out]
        n929 = control-ref of="queryThreat"() -> (w1622:refnum<vi>)
        n930 = call "Dropdown Selection (SubVI).vi"("reference"=w1622) -> ("element"=w1623:string)
        n931 = Format Into String(format string="SELECT  Experiment.Date, Shots.impact\nFROM Shots, Experiment where Shots.Expt = Experiment.expt\nand Experiment.Date Between #%s# And #%s# AND Experiment.threat Like '%%%s%%'\nORDER BY Experiment.Date" ("SQL statement"), error in=w1630, "beginCUSUM", "endCUSUM", w1623) -> (resulting string=w1621:string, error out=w1620:errorcluster)  [unwired: 1 in]
        n932 = call "Fetch Data (SubVI).vi"("error IN"=w1620, "connectString"=w1617, "query string"=w1621) -> ("error OUT"=w1619:errorcluster, "recordset data"=w1618:string[][])
        n933 = call "Get V50s (SubVI).vi"("recordset data"=w1618) -> ("V50 Array"=w1653:dbl[], "V50 Table"=→"v50 data":string[][], "lastVelocity"=w1635:dbl)
        "CUSUM_lastVel" <- w1635
        n934 = call <vilib>:"Std Deviation and Variance.vi"("X"=w1653, "Weighting (Sample)"=enum16{"Sample", "Population"}."Sample") -> ("mean"=w1651:dbl, "standard deviation"=w1652:dbl)  [unwired: 1 out]
        "Average Velocity" <- w1651
        "CUSUM_stdDev" <- w1652
        n935 = Array Size(array=w1653) -> (size(s)=w1642:i32)
        n936 = Subtract(x=w1651, y=w1635) -> (x-y=w1636:dbl)
        n937 = Absolute Value(x=w1636) -> (abs(x)=w1637:dbl)
        n938 = Multiply(x=3.0, y=w1652) -> (x*y=w1641:dbl)
        n939 = Divide(x=w1637, y=w1652) -> (x/y=w1648:dbl)
        n940 = Subtract(x=w1651, y=w1641) -> (x-y=w1644:dbl)
        n941 = Add(x=w1651, y=w1641) -> (x+y=w1643:dbl)
        n942 = Initialize Array(w1651, w1642) -> (w1624:dbl[])
        n943 = Initialize Array(w1644, w1642) -> (w1645:dbl[])
        n944 = Initialize Array(w1643, w1642) -> (w1646:dbl[])
        n945 = Format Into String(format string="%3.1f" ("Format String"), error in=w1619, w1648) -> (resulting string=w1647:string, error out=w1654:errorcluster)  [unwired: 1 in]
        n946 = Greater?(x=3.0, y=w1648) -> (0:→"In Control":bool)
        n947 = Build Array(w1653, w1624, w1645, w1646) -> (w1627:dbl[][])
        n948 = property on="In Control" class="Bool (strict)"(error in=w1654, "Boolean Text.Text"=w1647) -> (error out=w1655:errorcluster)  [unwired: 1 in, 1 out]
        n949 = Bundle(0.0, 1.0, w1627) -> (→"Previous V50 Data":cluster{dbl, dbl, dbl[][]})  [unwired: 1 in]
        n950 = call <vilib>:"Simple Error Handler.vi"("error in (no error)"=w1655) -> ()  [unwired: 4 in, 5 out]
      }
      event "SHOTS", "Sort by AVG": Value Change {
        n951 = event-data() -> ()  [unwired: 1 in, 6 out]
        n952 = local read "SHOTS"() -> (w1657:T5[])
        n953 = call "Update Shot Table.vi"("Sort by AVG"="Sort by AVG", "shot array"=w1657) -> ("shotTable OUT"=w1659:string[][])
        n954 = local write "Table of Shots"(w1659) -> ()
      }
      event "Layer_1.plyNum", "Layer_2.plyNum", "Layer_3.plyNum", "Layer_4.plyNum", "Layer_5.plyNum", "Layer_6.plyNum", "fabAttribs_1.ozPerYd2", "fabAttribs_2.ozPerYd2", "fabAttribs_3.ozPerYd2", "fabAttribs_4.ozPerYd2", "fabAttribs_5.ozPerYd2", "fabAttribs_6.ozPerYd2": Value Change {
        n955 = event-data() -> ()  [unwired: 1 in, 6 out]
        n956 = local read "Layer_1"() -> (w1666:T3)
        n957 = local read "Layer_2"() -> (w1665:T3)
        n958 = local read "Layer_3"() -> (w1664:T3)
        n959 = local read "Layer_4"() -> (w1663:T3)
        n960 = local read "Layer_5"() -> (w1662:T3)
        n961 = local read "Layer_6"() -> (w1661:T3)
        n962 = Build Array(w1666, w1665, w1664, w1663, w1662, w1661) -> (w1667:T13)
        n963 = local read "fabAttribs_1"() -> (w1669:T4)
        n964 = local read "fabAttribs_2"() -> (w1671:T4)
        n965 = local read "fabAttribs_3"() -> (w1672:T4)
        n966 = local read "fabAttribs_4"() -> (w1673:T4)
        n967 = local read "fabAttribs_5"() -> (w1674:T4)
        n968 = local read "fabAttribs_6"() -> (w1670:T4)
        n969 = Build Array(w1669, w1671, w1672, w1673, w1674, w1670) -> (w1668:T14)
        n970 = for {
          tunnel: w1667 -> [w1694] mode=indexing
          shift-right: [w1696] -> w1676
          shift-left: 0 -> [w1695]
          tunnel: [w1693] -> w1686 mode=indexing
          tunnel: w1668 -> [w1690] mode=indexing
          n971 = Unbundle By Name(w1690) -> ("ozPerYd2"=w1691:string)
          n972 = Unbundle By Name(w1694) -> ("plyNum"=w1692:i32)
          n973 = Scan From String(input string=w1691, default 1=sgl 0.0 ("default value 1")) -> (output 1=w1689:sgl)  [unwired: 3 in, 3 out]
          n974 = Add(x=w1695, y=w1692) -> (x+y=w1696:i32)
          n975 = To Single Precision Float(number=w1692) -> (single precision float=w1688:sgl)
          n976 = Multiply(x=w1688, y=w1689) -> (x*y=w1693:sgl)
        }
        "totalNumPlies" <- w1676
        n977 = Divide(x=w1686, y=sgl 144.0) -> (x/y=w1684:sgl[])
        n978 = Index Array(array=w1684) -> (element #1=→"fab1_totalWt":sgl, element #2=→"fab2_totalWt":sgl, element #3=→"fab3_totalWt":sgl, element #4=→"fab4_totalWt":sgl, element #5=→"fab5_totalWt":sgl, element #6=→"fab6_totalWt":sgl)  [unwired: 6 in]
        n979 = Add Array Elements(numeric array=w1684) -> (sum=→"totalBAW":sgl)
      }
      event "clayCalArray": Value Change {
        n980 = event-data() -> ()  [unwired: 1 in, 6 out]
        n981 = for {
          N: 5 -> [_]
          tunnel: "clayCalArray" -> [w1719] mode=indexing
          shift-right: [w1718] -> w1703
          shift-left: "" -> [w1716]
          shift-right: [w1713] -> w1699
          shift-left: i16[] [] -> [w1712]
          n982 = Greater Than 0?(x=w1719) -> (x > 0?=w1720:bool)
          n983 = case shown="False" w1720 {
            tunnel: w1719 -> [_ w1726]
            tunnel: ["##" ("clayCalib") w1728] -> w1717
            tunnel: w1716 -> [w1723 w1727]
            tunnel: [w1723 w1727] -> w1715
            tunnel: [w1721 w1725] -> w1713
            tunnel: w1712 -> [w1721 w1724]
            frame False {
            }
            frame True {
              n984 = Format Into String(w1726) -> (resulting string=w1728:string)  [unwired: 3 in, 1 out]
              n985 = Build Array (concatenate)(w1724, w1726) -> (w1725:i16[])
            }
          }
          n986 = Concatenate Strings(w1715, w1717, "-" ("string")) -> (w1718:string)
        }
        n987 = String Length(string=w1703) -> (length=w1704:i32)
        n988 = Add Array Elements(numeric array=w1699) -> (sum=w1710:i16)
        n989 = Array Size(array=w1699) -> (size(s)=w1711:i32)
        n990 = Decrement(x=w1704) -> (x-1=w1701:i32)
        n991 = To Single Precision Float(number=w1710) -> (single precision float=w1709:sgl)
        n992 = To Single Precision Float(number=w1711) -> (single precision float=w1708:sgl)
        n993 = String Subset(string=w1703, length (rest)=w1701) -> (substring=w1702:string)  [unwired: 1 in]
        n994 = Divide(x=w1709, y=w1708) -> (x/y=→"clayAverage":sgl)
        n995 = local write "clayCalib"(w1702) -> ()
      }
      event "getRecord": Value Change {
        n996 = event-data() -> ()  [unwired: 1 in, 6 out]
        n997 = local write "lookupRec"(TRUE ("lookupRec")) -> ()
      }
      event "Method": Value Change {
        n998 = event-data() -> ("CtlRef"=w1735:refnum<vi>)  [unwired: 1 in, 5 out]
        n999 = call "Dropdown Selection (SubVI).vi"("reference"=w1735) -> ("element"=w1734:string)
        n1000 = Equal?(x=w1734, y="V50") -> (x = y?=w1732:bool)
        n1001 = property on="minV50" class="DigNum (strict)"("Visible"=w1732) -> ()  [unwired: 2 in, 2 out]
      }
    }
  }
